vi "MICSD Wakeup RSSI.vi"(8 "error in":errorcluster, 9 "# of Average Points (20)":i32=20, 10 "RSSI Mode (Single)":enum16{"Single Reading", "Average, 20 Rdngs"}(ring), 11 "VISA Resource Name":refnum<visa-resource-name>) -> (0 "error out":errorcluster, 2 "Wakeup RSSI":i16, 3 "dup VISA Resource Name":refnum<visa-resource-name>)   [LabVIEW 2020]
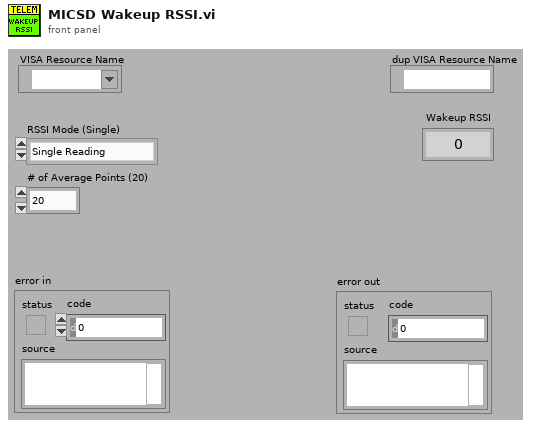
[diagram p1: front panel]
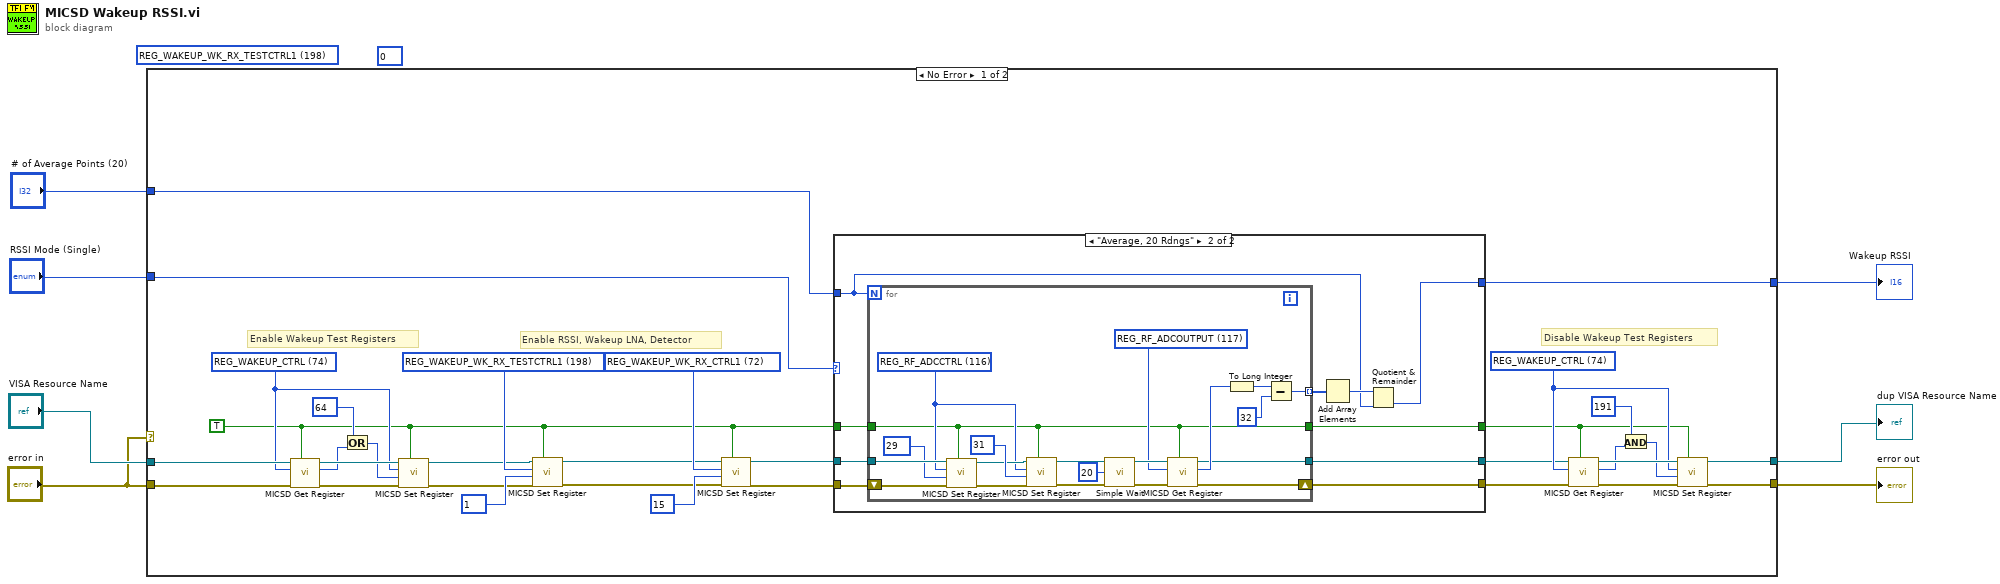
[diagram p0: block diagram]
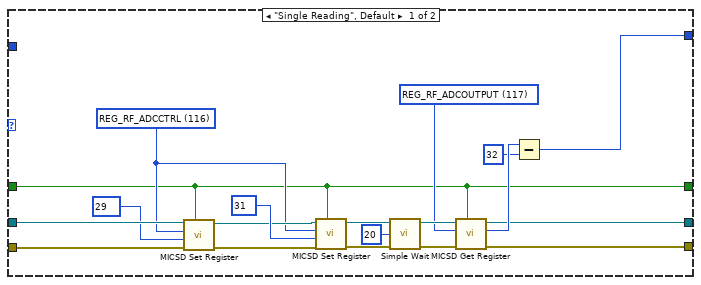
[diagram p2: hidden frame]
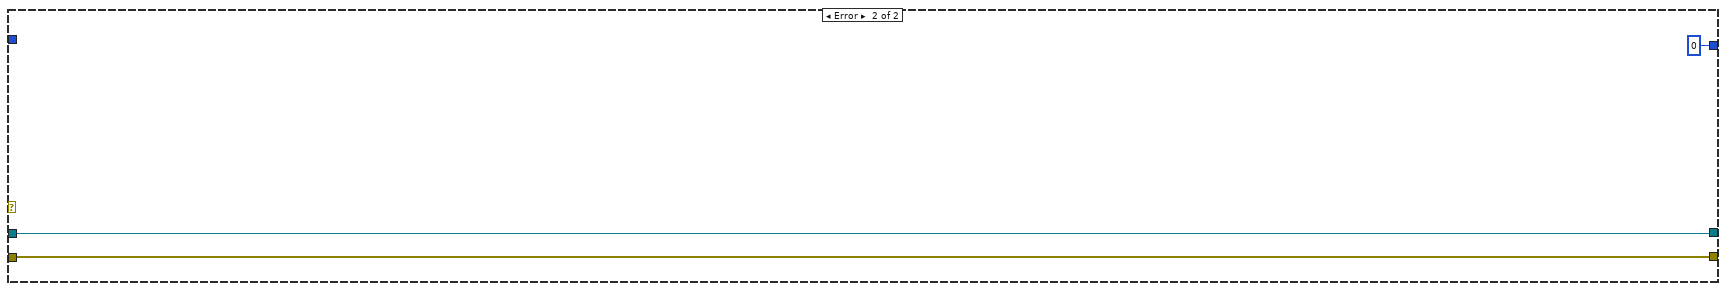
[diagram p3: hidden frame]
diagram:
  (unwired) u16 198 items=["---MANUAL ENTRY---"=1000, "REG_NOREG"=0, "REG_RXBUFF_USED"=1, "REG_RXBUFF_BSIZE"=2, "REG_TXBUFF_USED"=3, "REG_TXBUFF_BSIZE"=4, "REG_TXBUFF_MAXPACKSIZE"=5, "REG_MAC_ERRCLR"=6, "REG_MAC_TRAINNUM"=7, "REG_MAC_SYNCMATCH"=8, "REG_MAC_SYNC1"=9, "REG_MAC_SYNC2"=10, "REG_MAC_SYNC3"=11, "REG_MAC_SYNC4"=12, "REG_MAC_SYNC5"=13, "REG_MAC_MAXBERR"=14, "REG_MAC_ECCORR"=15, "REG_MAC_CRCERR"=16, "REG_MAC_BLKCNT1"=17, "REG_MAC_BLKCNT2"=18, "REG_MAC_IMDTRANSID1"=19, "REG_MAC_IMDTRANSID2"=20, "REG_MAC_IMDTRANSID3"=21, "REG_MAC_COMPANYID"=22, "REG_MAC_MODUSER"=23, "REG_MAC_CHANNEL"=25, "REG_MAC_CLEARWDOG"=26, "REG_MAC_CKCORRTHRESH"=27, "REG_HK_TXADDR"=28, "REG_HK_TXDATA"=29, "REG_HK_TXREPLY"=30, "REG_HK_USERDATA"=31, "REG_HK_USERSTATUS"=32, "REG_HK_LASTADDRESS"=33, "REG_HK_MODE"=34, "REG_MAC_STATUSSEQ"=35, "REG_MAC_MAXRETRIES"=36, "REG_MAC_RESENDTIME"=37, "REG_MAC_POWERSAVETIME"=38, "REG_MAC_HEAD_DET"=39, "REG_MAC_CTRL"=41, "REG_MAC_INITCOM"=42, "REG_INTERFACE_MODE"=43, "REG_TXRXBUFF_BOTH"=44, "REG_TXRXBUFF"=45, "REG_IRQ_RAWSTATUS1"=46, "REG_IRQ_ENABLE1"=47, "REG_IRQ_ENABLESET1"=48, "REG_IRQ_ENABLECLEAR1"=49, "REG_IRQ_RAWSTATUS2"=50, "REG_IRQ_ENABLE2"=51, "REG_IRQ_ENABLESET2"=52, "REG_IRQ_ENABLECLEAR2"=53, "REG_IRQ_STATUS1"=54, "REG_IRQ_STATUS2"=55, "REG_IRQ_AUXSTATUS"=56, "REG_TXBUFF_OVERFLOW"=57, "REG_PO0"=58, "REG_P01"=59, "REG_P02"=60, "REG_P03"=61, "REG_GP0"=62, "REG_GPI"=63, "REG_WAKEUP_245IN"=64, "REG_WAKEUP_COMPANYID"=65, "REG_WAKEUP_IMDTRANSID1"=66, "REG_WAKEUP_IMDTRANSID2"=67, "REG_WAKEUP_IMDTRANSID3"=68, "REG_WAKEUP_CHANNEL"=69, "REG_WAKEUP_MODUSER"=70, "REG_WAKEUP_DEVICEMODE"=71, "REG_WAKEUP_WK_RX_CTRL1"=72, "REG_WAKEUP_STACK_ADDR"=73, "REG_WAKEUP_CTRL"=74, "REG_WAKEUP_STROSCRTRIM"=75, "REG_WAKEUP_BIASTRIM"=76, "REG_WAKEUP_ANT245TUNE"=77, "REG_WAKEUP_WK_RX_RTRIMDET"=78, "REG_WAKEUP_WK_RX_RTRIMDEMOD"=79, "REG_WAKEUP_WK_RX_RSSIGAIN"=80, "REG_WAKEUP_LNAFREQ1"=81, "REG_WAKEUP_STACK"=83, "REG_WAKUP_XOSU"=84, "REG_WAKUP_CNTDROPOUT"=85, "REG_WAKEUP_CRCCTRL"=86, "REG_WAKEUP_CRCWORD1"=87, "REG_WAKEUP_CRCWORD2"=88, "REG_WAKEUP_WK_RX_CTRIM"=89, "REG_WAKEUP_VDDATRIM"=90, "REG_WAKEUP_VDDDTRIM"=91, "REG_WAKEUP_TESTIOBUFEN"=92, "REG_WAKEUP_TESTIOCLAMP"=93, "CORE_RESET_ADDRESS"=94, "CHIP_RESET_ADDRESS"=95, "REG_RF_TXGENCTRL"=96, "REG_RF_TXIFCTRL"=97, "REG_RF_TXRF_SEL_CTRL"=98, "REG_RF_TXRFPWRDEFAULTSET"=99, "REG_RF_RSSITRIM"=100, "REG_RF_TXIFOSCTUNE"=101, "REG_RF_TXIFGAINIMB"=102, "REG_RF_TXIFLOCK"=103, "REG_RF_RXRFLNAGAINTRIM"=104, "REG_RF_RXBIASTR"=105, "REG_RF_RXGENCTRL"=106, "REG_RF_RXIFADCDECLEV"=107, "REG_RF_RXIFDETFILTERTUNE"=108, "REG_RF_RXIFFILTERTUNE"=109, "REG_RF_GENENABLES"=110, "REG_RF_SYNTH_CHANNEL"=111, "REG_TX_RAMP_RTRIM"=112, "REG_TX_RAMP_CTRIM"=113, "REG_RF_XO_TRIM"=114, "REG_RF_SYNTH_SET_TRIM"=115, "REG_RF_ADCCTRL"=116, "REG_RF_ADCOUTPUT"=117, "REG_RF_TXIFAMP"=118, "REG_RF_SYNTH_RTRIM"=119, "REG_RF_SYNTH_CTRIM"=120, "REG_RF_SYNTH_CT"=121, "REG_RF_TXMIXER_IOSTRIM_HIGH_IP"=122, "REG_RF_TXMIXER_IOSTRIM_HIGH_IN"=123, "REG_RF_TXMIXER_IOSTRIM_HIGH_QP"=124, "REG_RF_TXMIXER_IOSTRIM_HIGH_QN"=125, "REG_HX_WUADDR"=126, "REG_REVISION"=127, "REG_NOREG_TEST"=128, "REG_DTEST_RXBUFF"=129, "REG_RXBUFF_NEXT_BLOCK"=130, "REG_RXBUFF_FIRST_IN_PACK"=131, "REG_RXBUFF_FIRST_EMPTY"=132, "REG_MAC_BYPASS"=133, "REG_DTEST_TXBUFF"=134, "REG_TXBUFF_NEXT_BLOCK"=135, "REG_TXBUFF_FIRST_IN_PACK"=136, "REG_TXBUFF_FIRST_EMPTY"=137, "REG_DTEST_SEQ"=138, "REG_DTEST_CKCORR"=139, "REG_MAC_TOPSTATE"=140, "REG_DTEST_INTERFACE"=141, "REG_IFACE_TXRX_BYPASS"=142, "REG_MAC_TXRXWAIT"=143, "REG_MAC_TXRFRAMP"=144, "REG_MAC_TRAINWORD"=145, "REG_MAC_TRAINWORD2"=146, "REG_MAC_SETTINGS"=147, "REG_MAC_CALSELECT1"=148, "REG_MAC_CALSELECT2"=149, "REG_MAC_ANTMATCHSEL"=150, "REG_MAC_ANTTUNESEL1"=151, "REG_MAC_ANTTUNESEL2"=152, "REG_MAC_ANTTUNESEL3"=153, "REG_MAC_ANTTUNESTEP"=154, "REG_MAC_WUMODEBURST"=156, "REG_MAC_WUOFFSHORT"=157, "REG_MAC_WUOFFLONG"=158, "REG_MAC_CLKRECCTRL"=159, "REG_HK_MODE_P2"=162, "REG_MAC_ANTTUNERES1"=164, "REG_MAC_ANTTUNERES2"=165, "REG_INTERFACE_MODE_TEST"=171, "REG_TXRXBUFF_BOTH_P2"=172, "REG_TXRXBUFF_P2"=173, "REG_IRQ_RAWSTATUS1_P2"=174, "REG_MAC_TXIFSTATUS1"=176, "REG_MAC_TXIFSTATUS2"=177, "REG_IRQ_RAWSTATUS2_P2"=178, "REG_MAC_TXIFRAMPDELAY"=179, "REG_MAC_TXIFRAMPSLOPE"=180, "REG_MAX_TXIFRAMP"=181, "REG_IRQ_STATUS1_P2"=182, "REG_IRQ_STATUS2_P2"=183, "REG_IRQ_AUXSTATUS_P2"=184, "REG_MAC_UNLOCK"=188, "REG_MAC_TXIFFREQ"=190, "REG_WAKEUP_TESTCTRL1"=192, "REG_WAKEUP_RX_EN_CNT"=193, "REG_WAKEUP_TESTENABLES"=194, "REG_WAKEUP_DTBI_CTRL"=195, "REG_WAKEUP_DTBO_CTRL"=196, "REG_WAKEUP_TESTIOBUFTEST"=197, "REG_WAKEUP_WK_RX_TESTCTRL1"=198, "REG_WAKEUP_WK_RX_TESTCTRL2"=199, "REG_WAKEUP_SENS_SEQUENCE_CTRL"=200, "REG_WAKEUP_LNABIAS"=201, "REG_WAKEUP_DET_TH_TRIM1"=202, "REG_WAKEUP_LNABIAS_NOM1"=203, "REG_WAKEUP_RX_TSHORT_TRIM1"=204, "REG_WAKEUP_LNABIAS_NOM2"=205, "REG_WAKEUP_RX_TLONG_TRIM1"=206, "REG_WAKEUP_LNA_NEGRTRIM_NOM1"=207, "REG_WAKEUP_RX_TBURST_TRIM1"=208, "REG_WAKEUP_RX_LNA_NEGRTRIM_NOM2"=209, "REG_WAKEUP_RX_BB_G_BW_SEL1"=210, "REG_WAKEUP_WK_RX_DET_IOSTRIM1"=212, "REG_WAKEUP_WK_RX_CTRL2"=214, "REG_WAKEUP_WK_RX_RSSIVOSTRIM"=215, "REG_WAKEUP_LNANEGR_EFF"=216, "REG_WAKEUP_XOSU_FAST"=217, "REG_WAKEUP_STROSCPWIDTH1"=218, "REG_WAKEUP_STROSCPERIOD1"=220, "REG_WAKEUP_STROSCPERIOD2"=221, "REG_WAKEUP_WK_RX_LNA_NEGRTRIM1"=222, "REG_RF_TXTESTENABLE"=224, "REG_RF_TXIFTESTMODE"=225, "REG_RF_RXTESTENABLE"=226, "REG_RF_RXIFTESTCTRL1"=227, "REG_RF_RXIFTESTCTRL2"=228, "REG_RF_RXIFTESTCTRL3"=229, "REG_RF_SYNTH_TESTCTRL1"=230, "REG_RF_SYNTH_TESTCTRL2"=231, "REG_RF_SYNTH_TESTCTRL3"=232, "REG_RF_ADCTEST1"=237, "REG_RF_ADCTEST2"=238, "REG_RF_TXMIXER_IOSTRIM_LOW_IP"=240, "REG_RF_TXMIXER_IOSTRIM_LOW_IN"=241, "REG_RF_TXMIXER_ISOTRIM_LOW_QP"=242, "REG_RF_TXMIXER_IOSTRIM_LOW_QN"=243, "REG_RF_SYNTH_KPD"=244, "REG_RF_SYNTH_LOLEV"=245, "REG_RF_TXRFPWRTUNEANTSET"=246, "REG_RF_TXPD_GAIN_CTRL"=247, "REG_RF_SYNTH_STARTUP"=248, "REG_RF_TXRFANTTUNE_TXMODE"=249, "REG_RF_TXRFANTTUNE_RXMODE"=250, "REG_RF_RXRFANTTUNE_TXMODE"=251, "REG_RF_RXRFANTTUNE_RXMODE"=252, "REG_ANTMATCH1"=253, "REG_ANTMATCH2"=254, "REG_REVISION_P2"=255] ("Register")
  (unwired) u8 0 ("Data")
  n1 = case shown="No Error" "error in" {
    tunnel: "VISA Resource Name" -> [w40 w90]
    tunnel: "error in" -> [w39 w89]
    tunnel: [w14 w89] -> w6
    tunnel: [w13 w90] -> w5
    tunnel: "RSSI Mode (Single)" -> [w11 _]
    tunnel: "# of Average Points (20)" -> [w9 _]
    tunnel: [w8 0] -> w1
    frame No Error {
      w12 = TRUE
      w15 = u16 74 items=["---MANUAL ENTRY---"=1000, "REG_NOREG"=0, "REG_RXBUFF_USED"=1, "REG_RXBUFF_BSIZE"=2, "REG_TXBUFF_USED"=3, "REG_TXBUFF_BSIZE"=4, "REG_TXBUFF_MAXPACKSIZE"=5, "REG_MAC_ERRCLR"=6, "REG_MAC_TRAINNUM"=7, "REG_MAC_SYNCMATCH"=8, "REG_MAC_SYNC1"=9, "REG_MAC_SYNC2"=10, "REG_MAC_SYNC3"=11, "REG_MAC_SYNC4"=12, "REG_MAC_SYNC5"=13, "REG_MAC_MAXBERR"=14, "REG_MAC_ECCORR"=15, "REG_MAC_CRCERR"=16, "REG_MAC_BLKCNT1"=17, "REG_MAC_BLKCNT2"=18, "REG_MAC_IMDTRANSID1"=19, "REG_MAC_IMDTRANSID2"=20, "REG_MAC_IMDTRANSID3"=21, "REG_MAC_COMPANYID"=22, "REG_MAC_MODUSER"=23, "REG_MAC_CHANNEL"=25, "REG_MAC_CLEARWDOG"=26, "REG_MAC_CKCORRTHRESH"=27, "REG_HK_TXADDR"=28, "REG_HK_TXDATA"=29, "REG_HK_TXREPLY"=30, "REG_HK_USERDATA"=31, "REG_HK_USERSTATUS"=32, "REG_HK_LASTADDRESS"=33, "REG_HK_MODE"=34, "REG_MAC_STATUSSEQ"=35, "REG_MAC_MAXRETRIES"=36, "REG_MAC_RESENDTIME"=37, "REG_MAC_POWERSAVETIME"=38, "REG_MAC_HEAD_DET"=39, "REG_MAC_CTRL"=41, "REG_MAC_INITCOM"=42, "REG_INTERFACE_MODE"=43, "REG_TXRXBUFF_BOTH"=44, "REG_TXRXBUFF"=45, "REG_IRQ_RAWSTATUS1"=46, "REG_IRQ_ENABLE1"=47, "REG_IRQ_ENABLESET1"=48, "REG_IRQ_ENABLECLEAR1"=49, "REG_IRQ_RAWSTATUS2"=50, "REG_IRQ_ENABLE2"=51, "REG_IRQ_ENABLESET2"=52, "REG_IRQ_ENABLECLEAR2"=53, "REG_IRQ_STATUS1"=54, "REG_IRQ_STATUS2"=55, "REG_IRQ_AUXSTATUS"=56, "REG_TXBUFF_OVERFLOW"=57, "REG_PO0"=58, "REG_P01"=59, "REG_P02"=60, "REG_P03"=61, "REG_GP0"=62, "REG_GPI"=63, "REG_WAKEUP_245IN"=64, "REG_WAKEUP_COMPANYID"=65, "REG_WAKEUP_IMDTRANSID1"=66, "REG_WAKEUP_IMDTRANSID2"=67, "REG_WAKEUP_IMDTRANSID3"=68, "REG_WAKEUP_CHANNEL"=69, "REG_WAKEUP_MODUSER"=70, "REG_WAKEUP_DEVICEMODE"=71, "REG_WAKEUP_WK_RX_CTRL1"=72, "REG_WAKEUP_STACK_ADDR"=73, "REG_WAKEUP_CTRL"=74, "REG_WAKEUP_STROSCRTRIM"=75, "REG_WAKEUP_BIASTRIM"=76, "REG_WAKEUP_ANT245TUNE"=77, "REG_WAKEUP_WK_RX_RTRIMDET"=78, "REG_WAKEUP_WK_RX_RTRIMDEMOD"=79, "REG_WAKEUP_WK_RX_RSSIGAIN"=80, "REG_WAKEUP_LNAFREQ1"=81, "REG_WAKEUP_STACK"=83, "REG_WAKUP_XOSU"=84, "REG_WAKUP_CNTDROPOUT"=85, "REG_WAKEUP_CRCCTRL"=86, "REG_WAKEUP_CRCWORD1"=87, "REG_WAKEUP_CRCWORD2"=88, "REG_WAKEUP_WK_RX_CTRIM"=89, "REG_WAKEUP_VDDATRIM"=90, "REG_WAKEUP_VDDDTRIM"=91, "REG_WAKEUP_TESTIOBUFEN"=92, "REG_WAKEUP_TESTIOCLAMP"=93, "CORE_RESET_ADDRESS"=94, "CHIP_RESET_ADDRESS"=95, "REG_RF_TXGENCTRL"=96, "REG_RF_TXIFCTRL"=97, "REG_RF_TXRF_SEL_CTRL"=98, "REG_RF_TXRFPWRDEFAULTSET"=99, "REG_RF_RSSITRIM"=100, "REG_RF_TXIFOSCTUNE"=101, "REG_RF_TXIFGAINIMB"=102, "REG_RF_TXIFLOCK"=103, "REG_RF_RXRFLNAGAINTRIM"=104, "REG_RF_RXBIASTR"=105, "REG_RF_RXGENCTRL"=106, "REG_RF_RXIFADCDECLEV"=107, "REG_RF_RXIFDETFILTERTUNE"=108, "REG_RF_RXIFFILTERTUNE"=109, "REG_RF_GENENABLES"=110, "REG_RF_SYNTH_CHANNEL"=111, "REG_TX_RAMP_RTRIM"=112, "REG_TX_RAMP_CTRIM"=113, "REG_RF_XO_TRIM"=114, "REG_RF_SYNTH_SET_TRIM"=115, "REG_RF_ADCCTRL"=116, "REG_RF_ADCOUTPUT"=117, "REG_RF_TXIFAMP"=118, "REG_RF_SYNTH_RTRIM"=119, "REG_RF_SYNTH_CTRIM"=120, "REG_RF_SYNTH_CT"=121, "REG_RF_TXMIXER_IOSTRIM_HIGH_IP"=122, "REG_RF_TXMIXER_IOSTRIM_HIGH_IN"=123, "REG_RF_TXMIXER_IOSTRIM_HIGH_QP"=124, "REG_RF_TXMIXER_IOSTRIM_HIGH_QN"=125, "REG_HX_WUADDR"=126, "REG_REVISION"=127, "REG_NOREG_TEST"=128, "REG_DTEST_RXBUFF"=129, "REG_RXBUFF_NEXT_BLOCK"=130, "REG_RXBUFF_FIRST_IN_PACK"=131, "REG_RXBUFF_FIRST_EMPTY"=132, "REG_MAC_BYPASS"=133, "REG_DTEST_TXBUFF"=134, "REG_TXBUFF_NEXT_BLOCK"=135, "REG_TXBUFF_FIRST_IN_PACK"=136, "REG_TXBUFF_FIRST_EMPTY"=137, "REG_DTEST_SEQ"=138, "REG_DTEST_CKCORR"=139, "REG_MAC_TOPSTATE"=140, "REG_DTEST_INTERFACE"=141, "REG_IFACE_TXRX_BYPASS"=142, "REG_MAC_TXRXWAIT"=143, "REG_MAC_TXRFRAMP"=144, "REG_MAC_TRAINWORD"=145, "REG_MAC_TRAINWORD2"=146, "REG_MAC_SETTINGS"=147, "REG_MAC_CALSELECT1"=148, "REG_MAC_CALSELECT2"=149, "REG_MAC_ANTMATCHSEL"=150, "REG_MAC_ANTTUNESEL1"=151, "REG_MAC_ANTTUNESEL2"=152, "REG_MAC_ANTTUNESEL3"=153, "REG_MAC_ANTTUNESTEP"=154, "REG_MAC_WUMODEBURST"=156, "REG_MAC_WUOFFSHORT"=157, "REG_MAC_WUOFFLONG"=158, "REG_MAC_CLKRECCTRL"=159, "REG_HK_MODE_P2"=162, "REG_MAC_ANTTUNERES1"=164, "REG_MAC_ANTTUNERES2"=165, "REG_INTERFACE_MODE_TEST"=171, "REG_TXRXBUFF_BOTH_P2"=172, "REG_TXRXBUFF_P2"=173, "REG_IRQ_RAWSTATUS1_P2"=174, "REG_MAC_TXIFSTATUS1"=176, "REG_MAC_TXIFSTATUS2"=177, "REG_IRQ_RAWSTATUS2_P2"=178, "REG_MAC_TXIFRAMPDELAY"=179, "REG_MAC_TXIFRAMPSLOPE"=180, "REG_MAX_TXIFRAMP"=181, "REG_IRQ_STATUS1_P2"=182, "REG_IRQ_STATUS2_P2"=183, "REG_IRQ_AUXSTATUS_P2"=184, "REG_MAC_UNLOCK"=188, "REG_MAC_TXIFFREQ"=190, "REG_WAKEUP_TESTCTRL1"=192, "REG_WAKEUP_RX_EN_CNT"=193, "REG_WAKEUP_TESTENABLES"=194, "REG_WAKEUP_DTBI_CTRL"=195, "REG_WAKEUP_DTBO_CTRL"=196, "REG_WAKEUP_TESTIOBUFTEST"=197, "REG_WAKEUP_WK_RX_TESTCTRL1"=198, "REG_WAKEUP_WK_RX_TESTCTRL2"=199, "REG_WAKEUP_SENS_SEQUENCE_CTRL"=200, "REG_WAKEUP_LNABIAS"=201, "REG_WAKEUP_DET_TH_TRIM1"=202, "REG_WAKEUP_LNABIAS_NOM1"=203, "REG_WAKEUP_RX_TSHORT_TRIM1"=204, "REG_WAKEUP_LNABIAS_NOM2"=205, "REG_WAKEUP_RX_TLONG_TRIM1"=206, "REG_WAKEUP_LNA_NEGRTRIM_NOM1"=207, "REG_WAKEUP_RX_TBURST_TRIM1"=208, "REG_WAKEUP_RX_LNA_NEGRTRIM_NOM2"=209, "REG_WAKEUP_RX_BB_G_BW_SEL1"=210, "REG_WAKEUP_WK_RX_DET_IOSTRIM1"=212, "REG_WAKEUP_WK_RX_CTRL2"=214, "REG_WAKEUP_WK_RX_RSSIVOSTRIM"=215, "REG_WAKEUP_LNANEGR_EFF"=216, "REG_WAKEUP_XOSU_FAST"=217, "REG_WAKEUP_STROSCPWIDTH1"=218, "REG_WAKEUP_STROSCPERIOD1"=220, "REG_WAKEUP_STROSCPERIOD2"=221, "REG_WAKEUP_WK_RX_LNA_NEGRTRIM1"=222, "REG_RF_TXTESTENABLE"=224, "REG_RF_TXIFTESTMODE"=225, "REG_RF_RXTESTENABLE"=226, "REG_RF_RXIFTESTCTRL1"=227, "REG_RF_RXIFTESTCTRL2"=228, "REG_RF_RXIFTESTCTRL3"=229, "REG_RF_SYNTH_TESTCTRL1"=230, "REG_RF_SYNTH_TESTCTRL2"=231, "REG_RF_SYNTH_TESTCTRL3"=232, "REG_RF_ADCTEST1"=237, "REG_RF_ADCTEST2"=238, "REG_RF_TXMIXER_IOSTRIM_LOW_IP"=240, "REG_RF_TXMIXER_IOSTRIM_LOW_IN"=241, "REG_RF_TXMIXER_ISOTRIM_LOW_QP"=242, "REG_RF_TXMIXER_IOSTRIM_LOW_QN"=243, "REG_RF_SYNTH_KPD"=244, "REG_RF_SYNTH_LOLEV"=245, "REG_RF_TXRFPWRTUNEANTSET"=246, "REG_RF_TXPD_GAIN_CTRL"=247, "REG_RF_SYNTH_STARTUP"=248, "REG_RF_TXRFANTTUNE_TXMODE"=249, "REG_RF_TXRFANTTUNE_RXMODE"=250, "REG_RF_RXRFANTTUNE_TXMODE"=251, "REG_RF_RXRFANTTUNE_RXMODE"=252, "REG_ANTMATCH1"=253, "REG_ANTMATCH2"=254, "REG_REVISION_P2"=255] ("Register")
      w26 = u16 72 items=["---MANUAL ENTRY---"=1000, "REG_NOREG"=0, "REG_RXBUFF_USED"=1, "REG_RXBUFF_BSIZE"=2, "REG_TXBUFF_USED"=3, "REG_TXBUFF_BSIZE"=4, "REG_TXBUFF_MAXPACKSIZE"=5, "REG_MAC_ERRCLR"=6, "REG_MAC_TRAINNUM"=7, "REG_MAC_SYNCMATCH"=8, "REG_MAC_SYNC1"=9, "REG_MAC_SYNC2"=10, "REG_MAC_SYNC3"=11, "REG_MAC_SYNC4"=12, "REG_MAC_SYNC5"=13, "REG_MAC_MAXBERR"=14, "REG_MAC_ECCORR"=15, "REG_MAC_CRCERR"=16, "REG_MAC_BLKCNT1"=17, "REG_MAC_BLKCNT2"=18, "REG_MAC_IMDTRANSID1"=19, "REG_MAC_IMDTRANSID2"=20, "REG_MAC_IMDTRANSID3"=21, "REG_MAC_COMPANYID"=22, "REG_MAC_MODUSER"=23, "REG_MAC_CHANNEL"=25, "REG_MAC_CLEARWDOG"=26, "REG_MAC_CKCORRTHRESH"=27, "REG_HK_TXADDR"=28, "REG_HK_TXDATA"=29, "REG_HK_TXREPLY"=30, "REG_HK_USERDATA"=31, "REG_HK_USERSTATUS"=32, "REG_HK_LASTADDRESS"=33, "REG_HK_MODE"=34, "REG_MAC_STATUSSEQ"=35, "REG_MAC_MAXRETRIES"=36, "REG_MAC_RESENDTIME"=37, "REG_MAC_POWERSAVETIME"=38, "REG_MAC_HEAD_DET"=39, "REG_MAC_CTRL"=41, "REG_MAC_INITCOM"=42, "REG_INTERFACE_MODE"=43, "REG_TXRXBUFF_BOTH"=44, "REG_TXRXBUFF"=45, "REG_IRQ_RAWSTATUS1"=46, "REG_IRQ_ENABLE1"=47, "REG_IRQ_ENABLESET1"=48, "REG_IRQ_ENABLECLEAR1"=49, "REG_IRQ_RAWSTATUS2"=50, "REG_IRQ_ENABLE2"=51, "REG_IRQ_ENABLESET2"=52, "REG_IRQ_ENABLECLEAR2"=53, "REG_IRQ_STATUS1"=54, "REG_IRQ_STATUS2"=55, "REG_IRQ_AUXSTATUS"=56, "REG_TXBUFF_OVERFLOW"=57, "REG_PO0"=58, "REG_P01"=59, "REG_P02"=60, "REG_P03"=61, "REG_GP0"=62, "REG_GPI"=63, "REG_WAKEUP_245IN"=64, "REG_WAKEUP_COMPANYID"=65, "REG_WAKEUP_IMDTRANSID1"=66, "REG_WAKEUP_IMDTRANSID2"=67, "REG_WAKEUP_IMDTRANSID3"=68, "REG_WAKEUP_CHANNEL"=69, "REG_WAKEUP_MODUSER"=70, "REG_WAKEUP_DEVICEMODE"=71, "REG_WAKEUP_WK_RX_CTRL1"=72, "REG_WAKEUP_STACK_ADDR"=73, "REG_WAKEUP_CTRL"=74, "REG_WAKEUP_STROSCRTRIM"=75, "REG_WAKEUP_BIASTRIM"=76, "REG_WAKEUP_ANT245TUNE"=77, "REG_WAKEUP_WK_RX_RTRIMDET"=78, "REG_WAKEUP_WK_RX_RTRIMDEMOD"=79, "REG_WAKEUP_WK_RX_RSSIGAIN"=80, "REG_WAKEUP_LNAFREQ1"=81, "REG_WAKEUP_STACK"=83, "REG_WAKUP_XOSU"=84, "REG_WAKUP_CNTDROPOUT"=85, "REG_WAKEUP_CRCCTRL"=86, "REG_WAKEUP_CRCWORD1"=87, "REG_WAKEUP_CRCWORD2"=88, "REG_WAKEUP_WK_RX_CTRIM"=89, "REG_WAKEUP_VDDATRIM"=90, "REG_WAKEUP_VDDDTRIM"=91, "REG_WAKEUP_TESTIOBUFEN"=92, "REG_WAKEUP_TESTIOCLAMP"=93, "CORE_RESET_ADDRESS"=94, "CHIP_RESET_ADDRESS"=95, "REG_RF_TXGENCTRL"=96, "REG_RF_TXIFCTRL"=97, "REG_RF_TXRF_SEL_CTRL"=98, "REG_RF_TXRFPWRDEFAULTSET"=99, "REG_RF_RSSITRIM"=100, "REG_RF_TXIFOSCTUNE"=101, "REG_RF_TXIFGAINIMB"=102, "REG_RF_TXIFLOCK"=103, "REG_RF_RXRFLNAGAINTRIM"=104, "REG_RF_RXBIASTR"=105, "REG_RF_RXGENCTRL"=106, "REG_RF_RXIFADCDECLEV"=107, "REG_RF_RXIFDETFILTERTUNE"=108, "REG_RF_RXIFFILTERTUNE"=109, "REG_RF_GENENABLES"=110, "REG_RF_SYNTH_CHANNEL"=111, "REG_TX_RAMP_RTRIM"=112, "REG_TX_RAMP_CTRIM"=113, "REG_RF_XO_TRIM"=114, "REG_RF_SYNTH_SET_TRIM"=115, "REG_RF_ADCCTRL"=116, "REG_RF_ADCOUTPUT"=117, "REG_RF_TXIFAMP"=118, "REG_RF_SYNTH_RTRIM"=119, "REG_RF_SYNTH_CTRIM"=120, "REG_RF_SYNTH_CT"=121, "REG_RF_TXMIXER_IOSTRIM_HIGH_IP"=122, "REG_RF_TXMIXER_IOSTRIM_HIGH_IN"=123, "REG_RF_TXMIXER_IOSTRIM_HIGH_QP"=124, "REG_RF_TXMIXER_IOSTRIM_HIGH_QN"=125, "REG_HX_WUADDR"=126, "REG_REVISION"=127, "REG_NOREG_TEST"=128, "REG_DTEST_RXBUFF"=129, "REG_RXBUFF_NEXT_BLOCK"=130, "REG_RXBUFF_FIRST_IN_PACK"=131, "REG_RXBUFF_FIRST_EMPTY"=132, "REG_MAC_BYPASS"=133, "REG_DTEST_TXBUFF"=134, "REG_TXBUFF_NEXT_BLOCK"=135, "REG_TXBUFF_FIRST_IN_PACK"=136, "REG_TXBUFF_FIRST_EMPTY"=137, "REG_DTEST_SEQ"=138, "REG_DTEST_CKCORR"=139, "REG_MAC_TOPSTATE"=140, "REG_DTEST_INTERFACE"=141, "REG_IFACE_TXRX_BYPASS"=142, "REG_MAC_TXRXWAIT"=143, "REG_MAC_TXRFRAMP"=144, "REG_MAC_TRAINWORD"=145, "REG_MAC_TRAINWORD2"=146, "REG_MAC_SETTINGS"=147, "REG_MAC_CALSELECT1"=148, "REG_MAC_CALSELECT2"=149, "REG_MAC_ANTMATCHSEL"=150, "REG_MAC_ANTTUNESEL1"=151, "REG_MAC_ANTTUNESEL2"=152, "REG_MAC_ANTTUNESEL3"=153, "REG_MAC_ANTTUNESTEP"=154, "REG_MAC_WUMODEBURST"=156, "REG_MAC_WUOFFSHORT"=157, "REG_MAC_WUOFFLONG"=158, "REG_MAC_CLKRECCTRL"=159, "REG_HK_MODE_P2"=162, "REG_MAC_ANTTUNERES1"=164, "REG_MAC_ANTTUNERES2"=165, "REG_INTERFACE_MODE_TEST"=171, "REG_TXRXBUFF_BOTH_P2"=172, "REG_TXRXBUFF_P2"=173, "REG_IRQ_RAWSTATUS1_P2"=174, "REG_MAC_TXIFSTATUS1"=176, "REG_MAC_TXIFSTATUS2"=177, "REG_IRQ_RAWSTATUS2_P2"=178, "REG_MAC_TXIFRAMPDELAY"=179, "REG_MAC_TXIFRAMPSLOPE"=180, "REG_MAX_TXIFRAMP"=181, "REG_IRQ_STATUS1_P2"=182, "REG_IRQ_STATUS2_P2"=183, "REG_IRQ_AUXSTATUS_P2"=184, "REG_MAC_UNLOCK"=188, "REG_MAC_TXIFFREQ"=190, "REG_WAKEUP_TESTCTRL1"=192, "REG_WAKEUP_RX_EN_CNT"=193, "REG_WAKEUP_TESTENABLES"=194, "REG_WAKEUP_DTBI_CTRL"=195, "REG_WAKEUP_DTBO_CTRL"=196, "REG_WAKEUP_TESTIOBUFTEST"=197, "REG_WAKEUP_WK_RX_TESTCTRL1"=198, "REG_WAKEUP_WK_RX_TESTCTRL2"=199, "REG_WAKEUP_SENS_SEQUENCE_CTRL"=200, "REG_WAKEUP_LNABIAS"=201, "REG_WAKEUP_DET_TH_TRIM1"=202, "REG_WAKEUP_LNABIAS_NOM1"=203, "REG_WAKEUP_RX_TSHORT_TRIM1"=204, "REG_WAKEUP_LNABIAS_NOM2"=205, "REG_WAKEUP_RX_TLONG_TRIM1"=206, "REG_WAKEUP_LNA_NEGRTRIM_NOM1"=207, "REG_WAKEUP_RX_TBURST_TRIM1"=208, "REG_WAKEUP_RX_LNA_NEGRTRIM_NOM2"=209, "REG_WAKEUP_RX_BB_G_BW_SEL1"=210, "REG_WAKEUP_WK_RX_DET_IOSTRIM1"=212, "REG_WAKEUP_WK_RX_CTRL2"=214, "REG_WAKEUP_WK_RX_RSSIVOSTRIM"=215, "REG_WAKEUP_LNANEGR_EFF"=216, "REG_WAKEUP_XOSU_FAST"=217, "REG_WAKEUP_STROSCPWIDTH1"=218, "REG_WAKEUP_STROSCPERIOD1"=220, "REG_WAKEUP_STROSCPERIOD2"=221, "REG_WAKEUP_WK_RX_LNA_NEGRTRIM1"=222, "REG_RF_TXTESTENABLE"=224, "REG_RF_TXIFTESTMODE"=225, "REG_RF_RXTESTENABLE"=226, "REG_RF_RXIFTESTCTRL1"=227, "REG_RF_RXIFTESTCTRL2"=228, "REG_RF_RXIFTESTCTRL3"=229, "REG_RF_SYNTH_TESTCTRL1"=230, "REG_RF_SYNTH_TESTCTRL2"=231, "REG_RF_SYNTH_TESTCTRL3"=232, "REG_RF_ADCTEST1"=237, "REG_RF_ADCTEST2"=238, "REG_RF_TXMIXER_IOSTRIM_LOW_IP"=240, "REG_RF_TXMIXER_IOSTRIM_LOW_IN"=241, "REG_RF_TXMIXER_ISOTRIM_LOW_QP"=242, "REG_RF_TXMIXER_IOSTRIM_LOW_QN"=243, "REG_RF_SYNTH_KPD"=244, "REG_RF_SYNTH_LOLEV"=245, "REG_RF_TXRFPWRTUNEANTSET"=246, "REG_RF_TXPD_GAIN_CTRL"=247, "REG_RF_SYNTH_STARTUP"=248, "REG_RF_TXRFANTTUNE_TXMODE"=249, "REG_RF_TXRFANTTUNE_RXMODE"=250, "REG_RF_RXRFANTTUNE_TXMODE"=251, "REG_RF_RXRFANTTUNE_RXMODE"=252, "REG_ANTMATCH1"=253, "REG_ANTMATCH2"=254, "REG_REVISION_P2"=255] ("Register")
      w28 = u16 198 items=["---MANUAL ENTRY---"=1000, "REG_NOREG"=0, "REG_RXBUFF_USED"=1, "REG_RXBUFF_BSIZE"=2, "REG_TXBUFF_USED"=3, "REG_TXBUFF_BSIZE"=4, "REG_TXBUFF_MAXPACKSIZE"=5, "REG_MAC_ERRCLR"=6, "REG_MAC_TRAINNUM"=7, "REG_MAC_SYNCMATCH"=8, "REG_MAC_SYNC1"=9, "REG_MAC_SYNC2"=10, "REG_MAC_SYNC3"=11, "REG_MAC_SYNC4"=12, "REG_MAC_SYNC5"=13, "REG_MAC_MAXBERR"=14, "REG_MAC_ECCORR"=15, "REG_MAC_CRCERR"=16, "REG_MAC_BLKCNT1"=17, "REG_MAC_BLKCNT2"=18, "REG_MAC_IMDTRANSID1"=19, "REG_MAC_IMDTRANSID2"=20, "REG_MAC_IMDTRANSID3"=21, "REG_MAC_COMPANYID"=22, "REG_MAC_MODUSER"=23, "REG_MAC_CHANNEL"=25, "REG_MAC_CLEARWDOG"=26, "REG_MAC_CKCORRTHRESH"=27, "REG_HK_TXADDR"=28, "REG_HK_TXDATA"=29, "REG_HK_TXREPLY"=30, "REG_HK_USERDATA"=31, "REG_HK_USERSTATUS"=32, "REG_HK_LASTADDRESS"=33, "REG_HK_MODE"=34, "REG_MAC_STATUSSEQ"=35, "REG_MAC_MAXRETRIES"=36, "REG_MAC_RESENDTIME"=37, "REG_MAC_POWERSAVETIME"=38, "REG_MAC_HEAD_DET"=39, "REG_MAC_CTRL"=41, "REG_MAC_INITCOM"=42, "REG_INTERFACE_MODE"=43, "REG_TXRXBUFF_BOTH"=44, "REG_TXRXBUFF"=45, "REG_IRQ_RAWSTATUS1"=46, "REG_IRQ_ENABLE1"=47, "REG_IRQ_ENABLESET1"=48, "REG_IRQ_ENABLECLEAR1"=49, "REG_IRQ_RAWSTATUS2"=50, "REG_IRQ_ENABLE2"=51, "REG_IRQ_ENABLESET2"=52, "REG_IRQ_ENABLECLEAR2"=53, "REG_IRQ_STATUS1"=54, "REG_IRQ_STATUS2"=55, "REG_IRQ_AUXSTATUS"=56, "REG_TXBUFF_OVERFLOW"=57, "REG_PO0"=58, "REG_P01"=59, "REG_P02"=60, "REG_P03"=61, "REG_GP0"=62, "REG_GPI"=63, "REG_WAKEUP_245IN"=64, "REG_WAKEUP_COMPANYID"=65, "REG_WAKEUP_IMDTRANSID1"=66, "REG_WAKEUP_IMDTRANSID2"=67, "REG_WAKEUP_IMDTRANSID3"=68, "REG_WAKEUP_CHANNEL"=69, "REG_WAKEUP_MODUSER"=70, "REG_WAKEUP_DEVICEMODE"=71, "REG_WAKEUP_WK_RX_CTRL1"=72, "REG_WAKEUP_STACK_ADDR"=73, "REG_WAKEUP_CTRL"=74, "REG_WAKEUP_STROSCRTRIM"=75, "REG_WAKEUP_BIASTRIM"=76, "REG_WAKEUP_ANT245TUNE"=77, "REG_WAKEUP_WK_RX_RTRIMDET"=78, "REG_WAKEUP_WK_RX_RTRIMDEMOD"=79, "REG_WAKEUP_WK_RX_RSSIGAIN"=80, "REG_WAKEUP_LNAFREQ1"=81, "REG_WAKEUP_STACK"=83, "REG_WAKUP_XOSU"=84, "REG_WAKUP_CNTDROPOUT"=85, "REG_WAKEUP_CRCCTRL"=86, "REG_WAKEUP_CRCWORD1"=87, "REG_WAKEUP_CRCWORD2"=88, "REG_WAKEUP_WK_RX_CTRIM"=89, "REG_WAKEUP_VDDATRIM"=90, "REG_WAKEUP_VDDDTRIM"=91, "REG_WAKEUP_TESTIOBUFEN"=92, "REG_WAKEUP_TESTIOCLAMP"=93, "CORE_RESET_ADDRESS"=94, "CHIP_RESET_ADDRESS"=95, "REG_RF_TXGENCTRL"=96, "REG_RF_TXIFCTRL"=97, "REG_RF_TXRF_SEL_CTRL"=98, "REG_RF_TXRFPWRDEFAULTSET"=99, "REG_RF_RSSITRIM"=100, "REG_RF_TXIFOSCTUNE"=101, "REG_RF_TXIFGAINIMB"=102, "REG_RF_TXIFLOCK"=103, "REG_RF_RXRFLNAGAINTRIM"=104, "REG_RF_RXBIASTR"=105, "REG_RF_RXGENCTRL"=106, "REG_RF_RXIFADCDECLEV"=107, "REG_RF_RXIFDETFILTERTUNE"=108, "REG_RF_RXIFFILTERTUNE"=109, "REG_RF_GENENABLES"=110, "REG_RF_SYNTH_CHANNEL"=111, "REG_TX_RAMP_RTRIM"=112, "REG_TX_RAMP_CTRIM"=113, "REG_RF_XO_TRIM"=114, "REG_RF_SYNTH_SET_TRIM"=115, "REG_RF_ADCCTRL"=116, "REG_RF_ADCOUTPUT"=117, "REG_RF_TXIFAMP"=118, "REG_RF_SYNTH_RTRIM"=119, "REG_RF_SYNTH_CTRIM"=120, "REG_RF_SYNTH_CT"=121, "REG_RF_TXMIXER_IOSTRIM_HIGH_IP"=122, "REG_RF_TXMIXER_IOSTRIM_HIGH_IN"=123, "REG_RF_TXMIXER_IOSTRIM_HIGH_QP"=124, "REG_RF_TXMIXER_IOSTRIM_HIGH_QN"=125, "REG_HX_WUADDR"=126, "REG_REVISION"=127, "REG_NOREG_TEST"=128, "REG_DTEST_RXBUFF"=129, "REG_RXBUFF_NEXT_BLOCK"=130, "REG_RXBUFF_FIRST_IN_PACK"=131, "REG_RXBUFF_FIRST_EMPTY"=132, "REG_MAC_BYPASS"=133, "REG_DTEST_TXBUFF"=134, "REG_TXBUFF_NEXT_BLOCK"=135, "REG_TXBUFF_FIRST_IN_PACK"=136, "REG_TXBUFF_FIRST_EMPTY"=137, "REG_DTEST_SEQ"=138, "REG_DTEST_CKCORR"=139, "REG_MAC_TOPSTATE"=140, "REG_DTEST_INTERFACE"=141, "REG_IFACE_TXRX_BYPASS"=142, "REG_MAC_TXRXWAIT"=143, "REG_MAC_TXRFRAMP"=144, "REG_MAC_TRAINWORD"=145, "REG_MAC_TRAINWORD2"=146, "REG_MAC_SETTINGS"=147, "REG_MAC_CALSELECT1"=148, "REG_MAC_CALSELECT2"=149, "REG_MAC_ANTMATCHSEL"=150, "REG_MAC_ANTTUNESEL1"=151, "REG_MAC_ANTTUNESEL2"=152, "REG_MAC_ANTTUNESEL3"=153, "REG_MAC_ANTTUNESTEP"=154, "REG_MAC_WUMODEBURST"=156, "REG_MAC_WUOFFSHORT"=157, "REG_MAC_WUOFFLONG"=158, "REG_MAC_CLKRECCTRL"=159, "REG_HK_MODE_P2"=162, "REG_MAC_ANTTUNERES1"=164, "REG_MAC_ANTTUNERES2"=165, "REG_INTERFACE_MODE_TEST"=171, "REG_TXRXBUFF_BOTH_P2"=172, "REG_TXRXBUFF_P2"=173, "REG_IRQ_RAWSTATUS1_P2"=174, "REG_MAC_TXIFSTATUS1"=176, "REG_MAC_TXIFSTATUS2"=177, "REG_IRQ_RAWSTATUS2_P2"=178, "REG_MAC_TXIFRAMPDELAY"=179, "REG_MAC_TXIFRAMPSLOPE"=180, "REG_MAX_TXIFRAMP"=181, "REG_IRQ_STATUS1_P2"=182, "REG_IRQ_STATUS2_P2"=183, "REG_IRQ_AUXSTATUS_P2"=184, "REG_MAC_UNLOCK"=188, "REG_MAC_TXIFFREQ"=190, "REG_WAKEUP_TESTCTRL1"=192, "REG_WAKEUP_RX_EN_CNT"=193, "REG_WAKEUP_TESTENABLES"=194, "REG_WAKEUP_DTBI_CTRL"=195, "REG_WAKEUP_DTBO_CTRL"=196, "REG_WAKEUP_TESTIOBUFTEST"=197, "REG_WAKEUP_WK_RX_TESTCTRL1"=198, "REG_WAKEUP_WK_RX_TESTCTRL2"=199, "REG_WAKEUP_SENS_SEQUENCE_CTRL"=200, "REG_WAKEUP_LNABIAS"=201, "REG_WAKEUP_DET_TH_TRIM1"=202, "REG_WAKEUP_LNABIAS_NOM1"=203, "REG_WAKEUP_RX_TSHORT_TRIM1"=204, "REG_WAKEUP_LNABIAS_NOM2"=205, "REG_WAKEUP_RX_TLONG_TRIM1"=206, "REG_WAKEUP_LNA_NEGRTRIM_NOM1"=207, "REG_WAKEUP_RX_TBURST_TRIM1"=208, "REG_WAKEUP_RX_LNA_NEGRTRIM_NOM2"=209, "REG_WAKEUP_RX_BB_G_BW_SEL1"=210, "REG_WAKEUP_WK_RX_DET_IOSTRIM1"=212, "REG_WAKEUP_WK_RX_CTRL2"=214, "REG_WAKEUP_WK_RX_RSSIVOSTRIM"=215, "REG_WAKEUP_LNANEGR_EFF"=216, "REG_WAKEUP_XOSU_FAST"=217, "REG_WAKEUP_STROSCPWIDTH1"=218, "REG_WAKEUP_STROSCPERIOD1"=220, "REG_WAKEUP_STROSCPERIOD2"=221, "REG_WAKEUP_WK_RX_LNA_NEGRTRIM1"=222, "REG_RF_TXTESTENABLE"=224, "REG_RF_TXIFTESTMODE"=225, "REG_RF_RXTESTENABLE"=226, "REG_RF_RXIFTESTCTRL1"=227, "REG_RF_RXIFTESTCTRL2"=228, "REG_RF_RXIFTESTCTRL3"=229, "REG_RF_SYNTH_TESTCTRL1"=230, "REG_RF_SYNTH_TESTCTRL2"=231, "REG_RF_SYNTH_TESTCTRL3"=232, "REG_RF_ADCTEST1"=237, "REG_RF_ADCTEST2"=238, "REG_RF_TXMIXER_IOSTRIM_LOW_IP"=240, "REG_RF_TXMIXER_IOSTRIM_LOW_IN"=241, "REG_RF_TXMIXER_ISOTRIM_LOW_QP"=242, "REG_RF_TXMIXER_IOSTRIM_LOW_QN"=243, "REG_RF_SYNTH_KPD"=244, "REG_RF_SYNTH_LOLEV"=245, "REG_RF_TXRFPWRTUNEANTSET"=246, "REG_RF_TXPD_GAIN_CTRL"=247, "REG_RF_SYNTH_STARTUP"=248, "REG_RF_TXRFANTTUNE_TXMODE"=249, "REG_RF_TXRFANTTUNE_RXMODE"=250, "REG_RF_RXRFANTTUNE_TXMODE"=251, "REG_RF_RXRFANTTUNE_RXMODE"=252, "REG_ANTMATCH1"=253, "REG_ANTMATCH2"=254, "REG_REVISION_P2"=255] ("Register")
      w33 = u16 74 items=["---MANUAL ENTRY---"=1000, "REG_NOREG"=0, "REG_RXBUFF_USED"=1, "REG_RXBUFF_BSIZE"=2, "REG_TXBUFF_USED"=3, "REG_TXBUFF_BSIZE"=4, "REG_TXBUFF_MAXPACKSIZE"=5, "REG_MAC_ERRCLR"=6, "REG_MAC_TRAINNUM"=7, "REG_MAC_SYNCMATCH"=8, "REG_MAC_SYNC1"=9, "REG_MAC_SYNC2"=10, "REG_MAC_SYNC3"=11, "REG_MAC_SYNC4"=12, "REG_MAC_SYNC5"=13, "REG_MAC_MAXBERR"=14, "REG_MAC_ECCORR"=15, "REG_MAC_CRCERR"=16, "REG_MAC_BLKCNT1"=17, "REG_MAC_BLKCNT2"=18, "REG_MAC_IMDTRANSID1"=19, "REG_MAC_IMDTRANSID2"=20, "REG_MAC_IMDTRANSID3"=21, "REG_MAC_COMPANYID"=22, "REG_MAC_MODUSER"=23, "REG_MAC_CHANNEL"=25, "REG_MAC_CLEARWDOG"=26, "REG_MAC_CKCORRTHRESH"=27, "REG_HK_TXADDR"=28, "REG_HK_TXDATA"=29, "REG_HK_TXREPLY"=30, "REG_HK_USERDATA"=31, "REG_HK_USERSTATUS"=32, "REG_HK_LASTADDRESS"=33, "REG_HK_MODE"=34, "REG_MAC_STATUSSEQ"=35, "REG_MAC_MAXRETRIES"=36, "REG_MAC_RESENDTIME"=37, "REG_MAC_POWERSAVETIME"=38, "REG_MAC_HEAD_DET"=39, "REG_MAC_CTRL"=41, "REG_MAC_INITCOM"=42, "REG_INTERFACE_MODE"=43, "REG_TXRXBUFF_BOTH"=44, "REG_TXRXBUFF"=45, "REG_IRQ_RAWSTATUS1"=46, "REG_IRQ_ENABLE1"=47, "REG_IRQ_ENABLESET1"=48, "REG_IRQ_ENABLECLEAR1"=49, "REG_IRQ_RAWSTATUS2"=50, "REG_IRQ_ENABLE2"=51, "REG_IRQ_ENABLESET2"=52, "REG_IRQ_ENABLECLEAR2"=53, "REG_IRQ_STATUS1"=54, "REG_IRQ_STATUS2"=55, "REG_IRQ_AUXSTATUS"=56, "REG_TXBUFF_OVERFLOW"=57, "REG_PO0"=58, "REG_P01"=59, "REG_P02"=60, "REG_P03"=61, "REG_GP0"=62, "REG_GPI"=63, "REG_WAKEUP_245IN"=64, "REG_WAKEUP_COMPANYID"=65, "REG_WAKEUP_IMDTRANSID1"=66, "REG_WAKEUP_IMDTRANSID2"=67, "REG_WAKEUP_IMDTRANSID3"=68, "REG_WAKEUP_CHANNEL"=69, "REG_WAKEUP_MODUSER"=70, "REG_WAKEUP_DEVICEMODE"=71, "REG_WAKEUP_WK_RX_CTRL1"=72, "REG_WAKEUP_STACK_ADDR"=73, "REG_WAKEUP_CTRL"=74, "REG_WAKEUP_STROSCRTRIM"=75, "REG_WAKEUP_BIASTRIM"=76, "REG_WAKEUP_ANT245TUNE"=77, "REG_WAKEUP_WK_RX_RTRIMDET"=78, "REG_WAKEUP_WK_RX_RTRIMDEMOD"=79, "REG_WAKEUP_WK_RX_RSSIGAIN"=80, "REG_WAKEUP_LNAFREQ1"=81, "REG_WAKEUP_STACK"=83, "REG_WAKUP_XOSU"=84, "REG_WAKUP_CNTDROPOUT"=85, "REG_WAKEUP_CRCCTRL"=86, "REG_WAKEUP_CRCWORD1"=87, "REG_WAKEUP_CRCWORD2"=88, "REG_WAKEUP_WK_RX_CTRIM"=89, "REG_WAKEUP_VDDATRIM"=90, "REG_WAKEUP_VDDDTRIM"=91, "REG_WAKEUP_TESTIOBUFEN"=92, "REG_WAKEUP_TESTIOCLAMP"=93, "CORE_RESET_ADDRESS"=94, "CHIP_RESET_ADDRESS"=95, "REG_RF_TXGENCTRL"=96, "REG_RF_TXIFCTRL"=97, "REG_RF_TXRF_SEL_CTRL"=98, "REG_RF_TXRFPWRDEFAULTSET"=99, "REG_RF_RSSITRIM"=100, "REG_RF_TXIFOSCTUNE"=101, "REG_RF_TXIFGAINIMB"=102, "REG_RF_TXIFLOCK"=103, "REG_RF_RXRFLNAGAINTRIM"=104, "REG_RF_RXBIASTR"=105, "REG_RF_RXGENCTRL"=106, "REG_RF_RXIFADCDECLEV"=107, "REG_RF_RXIFDETFILTERTUNE"=108, "REG_RF_RXIFFILTERTUNE"=109, "REG_RF_GENENABLES"=110, "REG_RF_SYNTH_CHANNEL"=111, "REG_TX_RAMP_RTRIM"=112, "REG_TX_RAMP_CTRIM"=113, "REG_RF_XO_TRIM"=114, "REG_RF_SYNTH_SET_TRIM"=115, "REG_RF_ADCCTRL"=116, "REG_RF_ADCOUTPUT"=117, "REG_RF_TXIFAMP"=118, "REG_RF_SYNTH_RTRIM"=119, "REG_RF_SYNTH_CTRIM"=120, "REG_RF_SYNTH_CT"=121, "REG_RF_TXMIXER_IOSTRIM_HIGH_IP"=122, "REG_RF_TXMIXER_IOSTRIM_HIGH_IN"=123, "REG_RF_TXMIXER_IOSTRIM_HIGH_QP"=124, "REG_RF_TXMIXER_IOSTRIM_HIGH_QN"=125, "REG_HX_WUADDR"=126, "REG_REVISION"=127, "REG_NOREG_TEST"=128, "REG_DTEST_RXBUFF"=129, "REG_RXBUFF_NEXT_BLOCK"=130, "REG_RXBUFF_FIRST_IN_PACK"=131, "REG_RXBUFF_FIRST_EMPTY"=132, "REG_MAC_BYPASS"=133, "REG_DTEST_TXBUFF"=134, "REG_TXBUFF_NEXT_BLOCK"=135, "REG_TXBUFF_FIRST_IN_PACK"=136, "REG_TXBUFF_FIRST_EMPTY"=137, "REG_DTEST_SEQ"=138, "REG_DTEST_CKCORR"=139, "REG_MAC_TOPSTATE"=140, "REG_DTEST_INTERFACE"=141, "REG_IFACE_TXRX_BYPASS"=142, "REG_MAC_TXRXWAIT"=143, "REG_MAC_TXRFRAMP"=144, "REG_MAC_TRAINWORD"=145, "REG_MAC_TRAINWORD2"=146, "REG_MAC_SETTINGS"=147, "REG_MAC_CALSELECT1"=148, "REG_MAC_CALSELECT2"=149, "REG_MAC_ANTMATCHSEL"=150, "REG_MAC_ANTTUNESEL1"=151, "REG_MAC_ANTTUNESEL2"=152, "REG_MAC_ANTTUNESEL3"=153, "REG_MAC_ANTTUNESTEP"=154, "REG_MAC_WUMODEBURST"=156, "REG_MAC_WUOFFSHORT"=157, "REG_MAC_WUOFFLONG"=158, "REG_MAC_CLKRECCTRL"=159, "REG_HK_MODE_P2"=162, "REG_MAC_ANTTUNERES1"=164, "REG_MAC_ANTTUNERES2"=165, "REG_INTERFACE_MODE_TEST"=171, "REG_TXRXBUFF_BOTH_P2"=172, "REG_TXRXBUFF_P2"=173, "REG_IRQ_RAWSTATUS1_P2"=174, "REG_MAC_TXIFSTATUS1"=176, "REG_MAC_TXIFSTATUS2"=177, "REG_IRQ_RAWSTATUS2_P2"=178, "REG_MAC_TXIFRAMPDELAY"=179, "REG_MAC_TXIFRAMPSLOPE"=180, "REG_MAX_TXIFRAMP"=181, "REG_IRQ_STATUS1_P2"=182, "REG_IRQ_STATUS2_P2"=183, "REG_IRQ_AUXSTATUS_P2"=184, "REG_MAC_UNLOCK"=188, "REG_MAC_TXIFFREQ"=190, "REG_WAKEUP_TESTCTRL1"=192, "REG_WAKEUP_RX_EN_CNT"=193, "REG_WAKEUP_TESTENABLES"=194, "REG_WAKEUP_DTBI_CTRL"=195, "REG_WAKEUP_DTBO_CTRL"=196, "REG_WAKEUP_TESTIOBUFTEST"=197, "REG_WAKEUP_WK_RX_TESTCTRL1"=198, "REG_WAKEUP_WK_RX_TESTCTRL2"=199, "REG_WAKEUP_SENS_SEQUENCE_CTRL"=200, "REG_WAKEUP_LNABIAS"=201, "REG_WAKEUP_DET_TH_TRIM1"=202, "REG_WAKEUP_LNABIAS_NOM1"=203, "REG_WAKEUP_RX_TSHORT_TRIM1"=204, "REG_WAKEUP_LNABIAS_NOM2"=205, "REG_WAKEUP_RX_TLONG_TRIM1"=206, "REG_WAKEUP_LNA_NEGRTRIM_NOM1"=207, "REG_WAKEUP_RX_TBURST_TRIM1"=208, "REG_WAKEUP_RX_LNA_NEGRTRIM_NOM2"=209, "REG_WAKEUP_RX_BB_G_BW_SEL1"=210, "REG_WAKEUP_WK_RX_DET_IOSTRIM1"=212, "REG_WAKEUP_WK_RX_CTRL2"=214, "REG_WAKEUP_WK_RX_RSSIVOSTRIM"=215, "REG_WAKEUP_LNANEGR_EFF"=216, "REG_WAKEUP_XOSU_FAST"=217, "REG_WAKEUP_STROSCPWIDTH1"=218, "REG_WAKEUP_STROSCPERIOD1"=220, "REG_WAKEUP_STROSCPERIOD2"=221, "REG_WAKEUP_WK_RX_LNA_NEGRTRIM1"=222, "REG_RF_TXTESTENABLE"=224, "REG_RF_TXIFTESTMODE"=225, "REG_RF_RXTESTENABLE"=226, "REG_RF_RXIFTESTCTRL1"=227, "REG_RF_RXIFTESTCTRL2"=228, "REG_RF_RXIFTESTCTRL3"=229, "REG_RF_SYNTH_TESTCTRL1"=230, "REG_RF_SYNTH_TESTCTRL2"=231, "REG_RF_SYNTH_TESTCTRL3"=232, "REG_RF_ADCTEST1"=237, "REG_RF_ADCTEST2"=238, "REG_RF_TXMIXER_IOSTRIM_LOW_IP"=240, "REG_RF_TXMIXER_IOSTRIM_LOW_IN"=241, "REG_RF_TXMIXER_ISOTRIM_LOW_QP"=242, "REG_RF_TXMIXER_IOSTRIM_LOW_QN"=243, "REG_RF_SYNTH_KPD"=244, "REG_RF_SYNTH_LOLEV"=245, "REG_RF_TXRFPWRTUNEANTSET"=246, "REG_RF_TXPD_GAIN_CTRL"=247, "REG_RF_SYNTH_STARTUP"=248, "REG_RF_TXRFANTTUNE_TXMODE"=249, "REG_RF_TXRFANTTUNE_RXMODE"=250, "REG_RF_RXRFANTTUNE_TXMODE"=251, "REG_RF_RXRFANTTUNE_RXMODE"=252, "REG_ANTMATCH1"=253, "REG_ANTMATCH2"=254, "REG_REVISION_P2"=255] ("Register")
      # "Enable RSSI, Wakeup LNA, Detector"
      # "Enable Wakeup Test Registers"
      # "Disable Wakeup Test Registers"
      n2 = call "MICSD Get Register.vi"("Execute on Remote?(F)"=w12, "error in (no error)"=w39, "Address"=w15, "VISA Resource Name"=w40) -> ("error out"=w20:errorcluster, "Data"=w18:u8, "dup VISA Resource Name"=w22:refnum<visa-resource-name>)  [unwired: 5 in]
      n3 = Or(x=u8 64 ("Data"), y=w18) -> (x .or. y?=w17:u8)
      n4 = call "MICSD Set Register.vi"("Execute on Remote?(F)"=w12, "error in (no error)"=w20, "Data"=w17, "Address"=w15, "VISA Resource Name"=w22) -> ("error out"=w19:errorcluster, "dup VISA Resource Name"=w21:refnum<visa-resource-name>)  [unwired: 5 in]
      n5 = call "MICSD Set Register.vi"("Execute on Remote?(F)"=w12, "error in (no error)"=w19, "Data"=u8 1, "Address"=w28, "VISA Resource Name"=w21) -> ("error out"=w23:errorcluster, "dup VISA Resource Name"=w24:refnum<visa-resource-name>)  [unwired: 5 in]
      n6 = call "MICSD Set Register.vi"("Execute on Remote?(F)"=w12, "error in (no error)"=w23, "Data"=u8 15, "Address"=w26, "VISA Resource Name"=w24) -> ("error out"=w30:errorcluster, "dup VISA Resource Name"=w29:refnum<visa-resource-name>)  [unwired: 5 in]
      n7 = case shown="\"Average, 20 Rdngs\"" w11 {
        tunnel: w29 -> [w55 w68]
        tunnel: w30 -> [w54 w67]
        tunnel: [w45 w66] -> w32
        tunnel: w12 -> [w42 w65]
        tunnel: [w44 w64] -> w31
        tunnel: w9 -> [_ w61]
        tunnel: [w42 w60] -> w10
        tunnel: [w41 w59] -> w8
        frame "Single Reading", Default {
          w47 = u16 117 items=["---MANUAL ENTRY---"=1000, "REG_NOREG"=0, "REG_RXBUFF_USED"=1, "REG_RXBUFF_BSIZE"=2, "REG_TXBUFF_USED"=3, "REG_TXBUFF_BSIZE"=4, "REG_TXBUFF_MAXPACKSIZE"=5, "REG_MAC_ERRCLR"=6, "REG_MAC_TRAINNUM"=7, "REG_MAC_SYNCMATCH"=8, "REG_MAC_SYNC1"=9, "REG_MAC_SYNC2"=10, "REG_MAC_SYNC3"=11, "REG_MAC_SYNC4"=12, "REG_MAC_SYNC5"=13, "REG_MAC_MAXBERR"=14, "REG_MAC_ECCORR"=15, "REG_MAC_CRCERR"=16, "REG_MAC_BLKCNT1"=17, "REG_MAC_BLKCNT2"=18, "REG_MAC_IMDTRANSID1"=19, "REG_MAC_IMDTRANSID2"=20, "REG_MAC_IMDTRANSID3"=21, "REG_MAC_COMPANYID"=22, "REG_MAC_MODUSER"=23, "REG_MAC_CHANNEL"=25, "REG_MAC_CLEARWDOG"=26, "REG_MAC_CKCORRTHRESH"=27, "REG_HK_TXADDR"=28, "REG_HK_TXDATA"=29, "REG_HK_TXREPLY"=30, "REG_HK_USERDATA"=31, "REG_HK_USERSTATUS"=32, "REG_HK_LASTADDRESS"=33, "REG_HK_MODE"=34, "REG_MAC_STATUSSEQ"=35, "REG_MAC_MAXRETRIES"=36, "REG_MAC_RESENDTIME"=37, "REG_MAC_POWERSAVETIME"=38, "REG_MAC_HEAD_DET"=39, "REG_MAC_CTRL"=41, "REG_MAC_INITCOM"=42, "REG_INTERFACE_MODE"=43, "REG_TXRXBUFF_BOTH"=44, "REG_TXRXBUFF"=45, "REG_IRQ_RAWSTATUS1"=46, "REG_IRQ_ENABLE1"=47, "REG_IRQ_ENABLESET1"=48, "REG_IRQ_ENABLECLEAR1"=49, "REG_IRQ_RAWSTATUS2"=50, "REG_IRQ_ENABLE2"=51, "REG_IRQ_ENABLESET2"=52, "REG_IRQ_ENABLECLEAR2"=53, "REG_IRQ_STATUS1"=54, "REG_IRQ_STATUS2"=55, "REG_IRQ_AUXSTATUS"=56, "REG_TXBUFF_OVERFLOW"=57, "REG_PO0"=58, "REG_P01"=59, "REG_P02"=60, "REG_P03"=61, "REG_GP0"=62, "REG_GPI"=63, "REG_WAKEUP_245IN"=64, "REG_WAKEUP_COMPANYID"=65, "REG_WAKEUP_IMDTRANSID1"=66, "REG_WAKEUP_IMDTRANSID2"=67, "REG_WAKEUP_IMDTRANSID3"=68, "REG_WAKEUP_CHANNEL"=69, "REG_WAKEUP_MODUSER"=70, "REG_WAKEUP_DEVICEMODE"=71, "REG_WAKEUP_WK_RX_CTRL1"=72, "REG_WAKEUP_STACK_ADDR"=73, "REG_WAKEUP_CTRL"=74, "REG_WAKEUP_STROSCRTRIM"=75, "REG_WAKEUP_BIASTRIM"=76, "REG_WAKEUP_ANT245TUNE"=77, "REG_WAKEUP_WK_RX_RTRIMDET"=78, "REG_WAKEUP_WK_RX_RTRIMDEMOD"=79, "REG_WAKEUP_WK_RX_RSSIGAIN"=80, "REG_WAKEUP_LNAFREQ1"=81, "REG_WAKEUP_STACK"=83, "REG_WAKUP_XOSU"=84, "REG_WAKUP_CNTDROPOUT"=85, "REG_WAKEUP_CRCCTRL"=86, "REG_WAKEUP_CRCWORD1"=87, "REG_WAKEUP_CRCWORD2"=88, "REG_WAKEUP_WK_RX_CTRIM"=89, "REG_WAKEUP_VDDATRIM"=90, "REG_WAKEUP_VDDDTRIM"=91, "REG_WAKEUP_TESTIOBUFEN"=92, "REG_WAKEUP_TESTIOCLAMP"=93, "CORE_RESET_ADDRESS"=94, "CHIP_RESET_ADDRESS"=95, "REG_RF_TXGENCTRL"=96, "REG_RF_TXIFCTRL"=97, "REG_RF_TXRF_SEL_CTRL"=98, "REG_RF_TXRFPWRDEFAULTSET"=99, "REG_RF_RSSITRIM"=100, "REG_RF_TXIFOSCTUNE"=101, "REG_RF_TXIFGAINIMB"=102, "REG_RF_TXIFLOCK"=103, "REG_RF_RXRFLNAGAINTRIM"=104, "REG_RF_RXBIASTR"=105, "REG_RF_RXGENCTRL"=106, "REG_RF_RXIFADCDECLEV"=107, "REG_RF_RXIFDETFILTERTUNE"=108, "REG_RF_RXIFFILTERTUNE"=109, "REG_RF_GENENABLES"=110, "REG_RF_SYNTH_CHANNEL"=111, "REG_TX_RAMP_RTRIM"=112, "REG_TX_RAMP_CTRIM"=113, "REG_RF_XO_TRIM"=114, "REG_RF_SYNTH_SET_TRIM"=115, "REG_RF_ADCCTRL"=116, "REG_RF_ADCOUTPUT"=117, "REG_RF_TXIFAMP"=118, "REG_RF_SYNTH_RTRIM"=119, "REG_RF_SYNTH_CTRIM"=120, "REG_RF_SYNTH_CT"=121, "REG_RF_TXMIXER_IOSTRIM_HIGH_IP"=122, "REG_RF_TXMIXER_IOSTRIM_HIGH_IN"=123, "REG_RF_TXMIXER_IOSTRIM_HIGH_QP"=124, "REG_RF_TXMIXER_IOSTRIM_HIGH_QN"=125, "REG_HX_WUADDR"=126, "REG_REVISION"=127, "REG_NOREG_TEST"=128, "REG_DTEST_RXBUFF"=129, "REG_RXBUFF_NEXT_BLOCK"=130, "REG_RXBUFF_FIRST_IN_PACK"=131, "REG_RXBUFF_FIRST_EMPTY"=132, "REG_MAC_BYPASS"=133, "REG_DTEST_TXBUFF"=134, "REG_TXBUFF_NEXT_BLOCK"=135, "REG_TXBUFF_FIRST_IN_PACK"=136, "REG_TXBUFF_FIRST_EMPTY"=137, "REG_DTEST_SEQ"=138, "REG_DTEST_CKCORR"=139, "REG_MAC_TOPSTATE"=140, "REG_DTEST_INTERFACE"=141, "REG_IFACE_TXRX_BYPASS"=142, "REG_MAC_TXRXWAIT"=143, "REG_MAC_TXRFRAMP"=144, "REG_MAC_TRAINWORD"=145, "REG_MAC_TRAINWORD2"=146, "REG_MAC_SETTINGS"=147, "REG_MAC_CALSELECT1"=148, "REG_MAC_CALSELECT2"=149, "REG_MAC_ANTMATCHSEL"=150, "REG_MAC_ANTTUNESEL1"=151, "REG_MAC_ANTTUNESEL2"=152, "REG_MAC_ANTTUNESEL3"=153, "REG_MAC_ANTTUNESTEP"=154, "REG_MAC_WUMODEBURST"=156, "REG_MAC_WUOFFSHORT"=157, "REG_MAC_WUOFFLONG"=158, "REG_MAC_CLKRECCTRL"=159, "REG_HK_MODE_P2"=162, "REG_MAC_ANTTUNERES1"=164, "REG_MAC_ANTTUNERES2"=165, "REG_INTERFACE_MODE_TEST"=171, "REG_TXRXBUFF_BOTH_P2"=172, "REG_TXRXBUFF_P2"=173, "REG_IRQ_RAWSTATUS1_P2"=174, "REG_MAC_TXIFSTATUS1"=176, "REG_MAC_TXIFSTATUS2"=177, "REG_IRQ_RAWSTATUS2_P2"=178, "REG_MAC_TXIFRAMPDELAY"=179, "REG_MAC_TXIFRAMPSLOPE"=180, "REG_MAX_TXIFRAMP"=181, "REG_IRQ_STATUS1_P2"=182, "REG_IRQ_STATUS2_P2"=183, "REG_IRQ_AUXSTATUS_P2"=184, "REG_MAC_UNLOCK"=188, "REG_MAC_TXIFFREQ"=190, "REG_WAKEUP_TESTCTRL1"=192, "REG_WAKEUP_RX_EN_CNT"=193, "REG_WAKEUP_TESTENABLES"=194, "REG_WAKEUP_DTBI_CTRL"=195, "REG_WAKEUP_DTBO_CTRL"=196, "REG_WAKEUP_TESTIOBUFTEST"=197, "REG_WAKEUP_WK_RX_TESTCTRL1"=198, "REG_WAKEUP_WK_RX_TESTCTRL2"=199, "REG_WAKEUP_SENS_SEQUENCE_CTRL"=200, "REG_WAKEUP_LNABIAS"=201, "REG_WAKEUP_DET_TH_TRIM1"=202, "REG_WAKEUP_LNABIAS_NOM1"=203, "REG_WAKEUP_RX_TSHORT_TRIM1"=204, "REG_WAKEUP_LNABIAS_NOM2"=205, "REG_WAKEUP_RX_TLONG_TRIM1"=206, "REG_WAKEUP_LNA_NEGRTRIM_NOM1"=207, "REG_WAKEUP_RX_TBURST_TRIM1"=208, "REG_WAKEUP_RX_LNA_NEGRTRIM_NOM2"=209, "REG_WAKEUP_RX_BB_G_BW_SEL1"=210, "REG_WAKEUP_WK_RX_DET_IOSTRIM1"=212, "REG_WAKEUP_WK_RX_CTRL2"=214, "REG_WAKEUP_WK_RX_RSSIVOSTRIM"=215, "REG_WAKEUP_LNANEGR_EFF"=216, "REG_WAKEUP_XOSU_FAST"=217, "REG_WAKEUP_STROSCPWIDTH1"=218, "REG_WAKEUP_STROSCPERIOD1"=220, "REG_WAKEUP_STROSCPERIOD2"=221, "REG_WAKEUP_WK_RX_LNA_NEGRTRIM1"=222, "REG_RF_TXTESTENABLE"=224, "REG_RF_TXIFTESTMODE"=225, "REG_RF_RXTESTENABLE"=226, "REG_RF_RXIFTESTCTRL1"=227, "REG_RF_RXIFTESTCTRL2"=228, "REG_RF_RXIFTESTCTRL3"=229, "REG_RF_SYNTH_TESTCTRL1"=230, "REG_RF_SYNTH_TESTCTRL2"=231, "REG_RF_SYNTH_TESTCTRL3"=232, "REG_RF_ADCTEST1"=237, "REG_RF_ADCTEST2"=238, "REG_RF_TXMIXER_IOSTRIM_LOW_IP"=240, "REG_RF_TXMIXER_IOSTRIM_LOW_IN"=241, "REG_RF_TXMIXER_ISOTRIM_LOW_QP"=242, "REG_RF_TXMIXER_IOSTRIM_LOW_QN"=243, "REG_RF_SYNTH_KPD"=244, "REG_RF_SYNTH_LOLEV"=245, "REG_RF_TXRFPWRTUNEANTSET"=246, "REG_RF_TXPD_GAIN_CTRL"=247, "REG_RF_SYNTH_STARTUP"=248, "REG_RF_TXRFANTTUNE_TXMODE"=249, "REG_RF_TXRFANTTUNE_RXMODE"=250, "REG_RF_RXRFANTTUNE_TXMODE"=251, "REG_RF_RXRFANTTUNE_RXMODE"=252, "REG_ANTMATCH1"=253, "REG_ANTMATCH2"=254, "REG_REVISION_P2"=255] ("Register")
          w52 = u16 116 items=["---MANUAL ENTRY---"=1000, "REG_NOREG"=0, "REG_RXBUFF_USED"=1, "REG_RXBUFF_BSIZE"=2, "REG_TXBUFF_USED"=3, "REG_TXBUFF_BSIZE"=4, "REG_TXBUFF_MAXPACKSIZE"=5, "REG_MAC_ERRCLR"=6, "REG_MAC_TRAINNUM"=7, "REG_MAC_SYNCMATCH"=8, "REG_MAC_SYNC1"=9, "REG_MAC_SYNC2"=10, "REG_MAC_SYNC3"=11, "REG_MAC_SYNC4"=12, "REG_MAC_SYNC5"=13, "REG_MAC_MAXBERR"=14, "REG_MAC_ECCORR"=15, "REG_MAC_CRCERR"=16, "REG_MAC_BLKCNT1"=17, "REG_MAC_BLKCNT2"=18, "REG_MAC_IMDTRANSID1"=19, "REG_MAC_IMDTRANSID2"=20, "REG_MAC_IMDTRANSID3"=21, "REG_MAC_COMPANYID"=22, "REG_MAC_MODUSER"=23, "REG_MAC_CHANNEL"=25, "REG_MAC_CLEARWDOG"=26, "REG_MAC_CKCORRTHRESH"=27, "REG_HK_TXADDR"=28, "REG_HK_TXDATA"=29, "REG_HK_TXREPLY"=30, "REG_HK_USERDATA"=31, "REG_HK_USERSTATUS"=32, "REG_HK_LASTADDRESS"=33, "REG_HK_MODE"=34, "REG_MAC_STATUSSEQ"=35, "REG_MAC_MAXRETRIES"=36, "REG_MAC_RESENDTIME"=37, "REG_MAC_POWERSAVETIME"=38, "REG_MAC_HEAD_DET"=39, "REG_MAC_CTRL"=41, "REG_MAC_INITCOM"=42, "REG_INTERFACE_MODE"=43, "REG_TXRXBUFF_BOTH"=44, "REG_TXRXBUFF"=45, "REG_IRQ_RAWSTATUS1"=46, "REG_IRQ_ENABLE1"=47, "REG_IRQ_ENABLESET1"=48, "REG_IRQ_ENABLECLEAR1"=49, "REG_IRQ_RAWSTATUS2"=50, "REG_IRQ_ENABLE2"=51, "REG_IRQ_ENABLESET2"=52, "REG_IRQ_ENABLECLEAR2"=53, "REG_IRQ_STATUS1"=54, "REG_IRQ_STATUS2"=55, "REG_IRQ_AUXSTATUS"=56, "REG_TXBUFF_OVERFLOW"=57, "REG_PO0"=58, "REG_P01"=59, "REG_P02"=60, "REG_P03"=61, "REG_GP0"=62, "REG_GPI"=63, "REG_WAKEUP_245IN"=64, "REG_WAKEUP_COMPANYID"=65, "REG_WAKEUP_IMDTRANSID1"=66, "REG_WAKEUP_IMDTRANSID2"=67, "REG_WAKEUP_IMDTRANSID3"=68, "REG_WAKEUP_CHANNEL"=69, "REG_WAKEUP_MODUSER"=70, "REG_WAKEUP_DEVICEMODE"=71, "REG_WAKEUP_WK_RX_CTRL1"=72, "REG_WAKEUP_STACK_ADDR"=73, "REG_WAKEUP_CTRL"=74, "REG_WAKEUP_STROSCRTRIM"=75, "REG_WAKEUP_BIASTRIM"=76, "REG_WAKEUP_ANT245TUNE"=77, "REG_WAKEUP_WK_RX_RTRIMDET"=78, "REG_WAKEUP_WK_RX_RTRIMDEMOD"=79, "REG_WAKEUP_WK_RX_RSSIGAIN"=80, "REG_WAKEUP_LNAFREQ1"=81, "REG_WAKEUP_STACK"=83, "REG_WAKUP_XOSU"=84, "REG_WAKUP_CNTDROPOUT"=85, "REG_WAKEUP_CRCCTRL"=86, "REG_WAKEUP_CRCWORD1"=87, "REG_WAKEUP_CRCWORD2"=88, "REG_WAKEUP_WK_RX_CTRIM"=89, "REG_WAKEUP_VDDATRIM"=90, "REG_WAKEUP_VDDDTRIM"=91, "REG_WAKEUP_TESTIOBUFEN"=92, "REG_WAKEUP_TESTIOCLAMP"=93, "CORE_RESET_ADDRESS"=94, "CHIP_RESET_ADDRESS"=95, "REG_RF_TXGENCTRL"=96, "REG_RF_TXIFCTRL"=97, "REG_RF_TXRF_SEL_CTRL"=98, "REG_RF_TXRFPWRDEFAULTSET"=99, "REG_RF_RSSITRIM"=100, "REG_RF_TXIFOSCTUNE"=101, "REG_RF_TXIFGAINIMB"=102, "REG_RF_TXIFLOCK"=103, "REG_RF_RXRFLNAGAINTRIM"=104, "REG_RF_RXBIASTR"=105, "REG_RF_RXGENCTRL"=106, "REG_RF_RXIFADCDECLEV"=107, "REG_RF_RXIFDETFILTERTUNE"=108, "REG_RF_RXIFFILTERTUNE"=109, "REG_RF_GENENABLES"=110, "REG_RF_SYNTH_CHANNEL"=111, "REG_TX_RAMP_RTRIM"=112, "REG_TX_RAMP_CTRIM"=113, "REG_RF_XO_TRIM"=114, "REG_RF_SYNTH_SET_TRIM"=115, "REG_RF_ADCCTRL"=116, "REG_RF_ADCOUTPUT"=117, "REG_RF_TXIFAMP"=118, "REG_RF_SYNTH_RTRIM"=119, "REG_RF_SYNTH_CTRIM"=120, "REG_RF_SYNTH_CT"=121, "REG_RF_TXMIXER_IOSTRIM_HIGH_IP"=122, "REG_RF_TXMIXER_IOSTRIM_HIGH_IN"=123, "REG_RF_TXMIXER_IOSTRIM_HIGH_QP"=124, "REG_RF_TXMIXER_IOSTRIM_HIGH_QN"=125, "REG_HX_WUADDR"=126, "REG_REVISION"=127, "REG_NOREG_TEST"=128, "REG_DTEST_RXBUFF"=129, "REG_RXBUFF_NEXT_BLOCK"=130, "REG_RXBUFF_FIRST_IN_PACK"=131, "REG_RXBUFF_FIRST_EMPTY"=132, "REG_MAC_BYPASS"=133, "REG_DTEST_TXBUFF"=134, "REG_TXBUFF_NEXT_BLOCK"=135, "REG_TXBUFF_FIRST_IN_PACK"=136, "REG_TXBUFF_FIRST_EMPTY"=137, "REG_DTEST_SEQ"=138, "REG_DTEST_CKCORR"=139, "REG_MAC_TOPSTATE"=140, "REG_DTEST_INTERFACE"=141, "REG_IFACE_TXRX_BYPASS"=142, "REG_MAC_TXRXWAIT"=143, "REG_MAC_TXRFRAMP"=144, "REG_MAC_TRAINWORD"=145, "REG_MAC_TRAINWORD2"=146, "REG_MAC_SETTINGS"=147, "REG_MAC_CALSELECT1"=148, "REG_MAC_CALSELECT2"=149, "REG_MAC_ANTMATCHSEL"=150, "REG_MAC_ANTTUNESEL1"=151, "REG_MAC_ANTTUNESEL2"=152, "REG_MAC_ANTTUNESEL3"=153, "REG_MAC_ANTTUNESTEP"=154, "REG_MAC_WUMODEBURST"=156, "REG_MAC_WUOFFSHORT"=157, "REG_MAC_WUOFFLONG"=158, "REG_MAC_CLKRECCTRL"=159, "REG_HK_MODE_P2"=162, "REG_MAC_ANTTUNERES1"=164, "REG_MAC_ANTTUNERES2"=165, "REG_INTERFACE_MODE_TEST"=171, "REG_TXRXBUFF_BOTH_P2"=172, "REG_TXRXBUFF_P2"=173, "REG_IRQ_RAWSTATUS1_P2"=174, "REG_MAC_TXIFSTATUS1"=176, "REG_MAC_TXIFSTATUS2"=177, "REG_IRQ_RAWSTATUS2_P2"=178, "REG_MAC_TXIFRAMPDELAY"=179, "REG_MAC_TXIFRAMPSLOPE"=180, "REG_MAX_TXIFRAMP"=181, "REG_IRQ_STATUS1_P2"=182, "REG_IRQ_STATUS2_P2"=183, "REG_IRQ_AUXSTATUS_P2"=184, "REG_MAC_UNLOCK"=188, "REG_MAC_TXIFFREQ"=190, "REG_WAKEUP_TESTCTRL1"=192, "REG_WAKEUP_RX_EN_CNT"=193, "REG_WAKEUP_TESTENABLES"=194, "REG_WAKEUP_DTBI_CTRL"=195, "REG_WAKEUP_DTBO_CTRL"=196, "REG_WAKEUP_TESTIOBUFTEST"=197, "REG_WAKEUP_WK_RX_TESTCTRL1"=198, "REG_WAKEUP_WK_RX_TESTCTRL2"=199, "REG_WAKEUP_SENS_SEQUENCE_CTRL"=200, "REG_WAKEUP_LNABIAS"=201, "REG_WAKEUP_DET_TH_TRIM1"=202, "REG_WAKEUP_LNABIAS_NOM1"=203, "REG_WAKEUP_RX_TSHORT_TRIM1"=204, "REG_WAKEUP_LNABIAS_NOM2"=205, "REG_WAKEUP_RX_TLONG_TRIM1"=206, "REG_WAKEUP_LNA_NEGRTRIM_NOM1"=207, "REG_WAKEUP_RX_TBURST_TRIM1"=208, "REG_WAKEUP_RX_LNA_NEGRTRIM_NOM2"=209, "REG_WAKEUP_RX_BB_G_BW_SEL1"=210, "REG_WAKEUP_WK_RX_DET_IOSTRIM1"=212, "REG_WAKEUP_WK_RX_CTRL2"=214, "REG_WAKEUP_WK_RX_RSSIVOSTRIM"=215, "REG_WAKEUP_LNANEGR_EFF"=216, "REG_WAKEUP_XOSU_FAST"=217, "REG_WAKEUP_STROSCPWIDTH1"=218, "REG_WAKEUP_STROSCPERIOD1"=220, "REG_WAKEUP_STROSCPERIOD2"=221, "REG_WAKEUP_WK_RX_LNA_NEGRTRIM1"=222, "REG_RF_TXTESTENABLE"=224, "REG_RF_TXIFTESTMODE"=225, "REG_RF_RXTESTENABLE"=226, "REG_RF_RXIFTESTCTRL1"=227, "REG_RF_RXIFTESTCTRL2"=228, "REG_RF_RXIFTESTCTRL3"=229, "REG_RF_SYNTH_TESTCTRL1"=230, "REG_RF_SYNTH_TESTCTRL2"=231, "REG_RF_SYNTH_TESTCTRL3"=232, "REG_RF_ADCTEST1"=237, "REG_RF_ADCTEST2"=238, "REG_RF_TXMIXER_IOSTRIM_LOW_IP"=240, "REG_RF_TXMIXER_IOSTRIM_LOW_IN"=241, "REG_RF_TXMIXER_ISOTRIM_LOW_QP"=242, "REG_RF_TXMIXER_IOSTRIM_LOW_QN"=243, "REG_RF_SYNTH_KPD"=244, "REG_RF_SYNTH_LOLEV"=245, "REG_RF_TXRFPWRTUNEANTSET"=246, "REG_RF_TXPD_GAIN_CTRL"=247, "REG_RF_SYNTH_STARTUP"=248, "REG_RF_TXRFANTTUNE_TXMODE"=249, "REG_RF_TXRFANTTUNE_RXMODE"=250, "REG_RF_RXRFANTTUNE_TXMODE"=251, "REG_RF_RXRFANTTUNE_RXMODE"=252, "REG_ANTMATCH1"=253, "REG_ANTMATCH2"=254, "REG_REVISION_P2"=255] ("Register")
          n8 = call "MICSD Set Register.vi"("Execute on Remote?(F)"=w42, "error in (no error)"=w54, "Data"=u8 29, "Address"=w52, "VISA Resource Name"=w55) -> ("error out"=w56:errorcluster, "dup VISA Resource Name"=w57:refnum<visa-resource-name>)  [unwired: 5 in]
          n9 = call "MICSD Set Register.vi"("Execute on Remote?(F)"=w42, "error in (no error)"=w56, "Data"=u8 31, "Address"=w52, "VISA Resource Name"=w57) -> ("error out"=w51:errorcluster, "dup VISA Resource Name"=w48:refnum<visa-resource-name>)  [unwired: 5 in]
          n10 = call "Simple Wait.vi"("mS"=u32 20, "error in"=w51) -> ("error out"=w49:errorcluster)  [unwired: 12 in, 1 out]
          n11 = call "MICSD Get Register.vi"("Execute on Remote?(F)"=w42, "error in (no error)"=w49, "Address"=w47, "VISA Resource Name"=w48) -> ("error out"=w45:errorcluster, "Data"=w46:u8, "dup VISA Resource Name"=w44:refnum<visa-resource-name>)  [unwired: 5 in]
          n12 = Subtract(x=w46, y=u8 32) -> (x-y=w41:u8)
        }
        frame "Average, 20 Rdngs" {
          n13 = for {
            N: w61 -> [_]
            tunnel: w68 -> [w84]
            tunnel: w65 -> [w69]
            tunnel: [w73] -> w64
            tunnel: [w72] -> w63 mode=indexing
            shift-right: [w74] -> w66
            shift-left: w67 -> [w83]
            tunnel: [w69] -> w60
            w76 = u16 117 items=["---MANUAL ENTRY---"=1000, "REG_NOREG"=0, "REG_RXBUFF_USED"=1, "REG_RXBUFF_BSIZE"=2, "REG_TXBUFF_USED"=3, "REG_TXBUFF_BSIZE"=4, "REG_TXBUFF_MAXPACKSIZE"=5, "REG_MAC_ERRCLR"=6, "REG_MAC_TRAINNUM"=7, "REG_MAC_SYNCMATCH"=8, "REG_MAC_SYNC1"=9, "REG_MAC_SYNC2"=10, "REG_MAC_SYNC3"=11, "REG_MAC_SYNC4"=12, "REG_MAC_SYNC5"=13, "REG_MAC_MAXBERR"=14, "REG_MAC_ECCORR"=15, "REG_MAC_CRCERR"=16, "REG_MAC_BLKCNT1"=17, "REG_MAC_BLKCNT2"=18, "REG_MAC_IMDTRANSID1"=19, "REG_MAC_IMDTRANSID2"=20, "REG_MAC_IMDTRANSID3"=21, "REG_MAC_COMPANYID"=22, "REG_MAC_MODUSER"=23, "REG_MAC_CHANNEL"=25, "REG_MAC_CLEARWDOG"=26, "REG_MAC_CKCORRTHRESH"=27, "REG_HK_TXADDR"=28, "REG_HK_TXDATA"=29, "REG_HK_TXREPLY"=30, "REG_HK_USERDATA"=31, "REG_HK_USERSTATUS"=32, "REG_HK_LASTADDRESS"=33, "REG_HK_MODE"=34, "REG_MAC_STATUSSEQ"=35, "REG_MAC_MAXRETRIES"=36, "REG_MAC_RESENDTIME"=37, "REG_MAC_POWERSAVETIME"=38, "REG_MAC_HEAD_DET"=39, "REG_MAC_CTRL"=41, "REG_MAC_INITCOM"=42, "REG_INTERFACE_MODE"=43, "REG_TXRXBUFF_BOTH"=44, "REG_TXRXBUFF"=45, "REG_IRQ_RAWSTATUS1"=46, "REG_IRQ_ENABLE1"=47, "REG_IRQ_ENABLESET1"=48, "REG_IRQ_ENABLECLEAR1"=49, "REG_IRQ_RAWSTATUS2"=50, "REG_IRQ_ENABLE2"=51, "REG_IRQ_ENABLESET2"=52, "REG_IRQ_ENABLECLEAR2"=53, "REG_IRQ_STATUS1"=54, "REG_IRQ_STATUS2"=55, "REG_IRQ_AUXSTATUS"=56, "REG_TXBUFF_OVERFLOW"=57, "REG_PO0"=58, "REG_P01"=59, "REG_P02"=60, "REG_P03"=61, "REG_GP0"=62, "REG_GPI"=63, "REG_WAKEUP_245IN"=64, "REG_WAKEUP_COMPANYID"=65, "REG_WAKEUP_IMDTRANSID1"=66, "REG_WAKEUP_IMDTRANSID2"=67, "REG_WAKEUP_IMDTRANSID3"=68, "REG_WAKEUP_CHANNEL"=69, "REG_WAKEUP_MODUSER"=70, "REG_WAKEUP_DEVICEMODE"=71, "REG_WAKEUP_WK_RX_CTRL1"=72, "REG_WAKEUP_STACK_ADDR"=73, "REG_WAKEUP_CTRL"=74, "REG_WAKEUP_STROSCRTRIM"=75, "REG_WAKEUP_BIASTRIM"=76, "REG_WAKEUP_ANT245TUNE"=77, "REG_WAKEUP_WK_RX_RTRIMDET"=78, "REG_WAKEUP_WK_RX_RTRIMDEMOD"=79, "REG_WAKEUP_WK_RX_RSSIGAIN"=80, "REG_WAKEUP_LNAFREQ1"=81, "REG_WAKEUP_STACK"=83, "REG_WAKUP_XOSU"=84, "REG_WAKUP_CNTDROPOUT"=85, "REG_WAKEUP_CRCCTRL"=86, "REG_WAKEUP_CRCWORD1"=87, "REG_WAKEUP_CRCWORD2"=88, "REG_WAKEUP_WK_RX_CTRIM"=89, "REG_WAKEUP_VDDATRIM"=90, "REG_WAKEUP_VDDDTRIM"=91, "REG_WAKEUP_TESTIOBUFEN"=92, "REG_WAKEUP_TESTIOCLAMP"=93, "CORE_RESET_ADDRESS"=94, "CHIP_RESET_ADDRESS"=95, "REG_RF_TXGENCTRL"=96, "REG_RF_TXIFCTRL"=97, "REG_RF_TXRF_SEL_CTRL"=98, "REG_RF_TXRFPWRDEFAULTSET"=99, "REG_RF_RSSITRIM"=100, "REG_RF_TXIFOSCTUNE"=101, "REG_RF_TXIFGAINIMB"=102, "REG_RF_TXIFLOCK"=103, "REG_RF_RXRFLNAGAINTRIM"=104, "REG_RF_RXBIASTR"=105, "REG_RF_RXGENCTRL"=106, "REG_RF_RXIFADCDECLEV"=107, "REG_RF_RXIFDETFILTERTUNE"=108, "REG_RF_RXIFFILTERTUNE"=109, "REG_RF_GENENABLES"=110, "REG_RF_SYNTH_CHANNEL"=111, "REG_TX_RAMP_RTRIM"=112, "REG_TX_RAMP_CTRIM"=113, "REG_RF_XO_TRIM"=114, "REG_RF_SYNTH_SET_TRIM"=115, "REG_RF_ADCCTRL"=116, "REG_RF_ADCOUTPUT"=117, "REG_RF_TXIFAMP"=118, "REG_RF_SYNTH_RTRIM"=119, "REG_RF_SYNTH_CTRIM"=120, "REG_RF_SYNTH_CT"=121, "REG_RF_TXMIXER_IOSTRIM_HIGH_IP"=122, "REG_RF_TXMIXER_IOSTRIM_HIGH_IN"=123, "REG_RF_TXMIXER_IOSTRIM_HIGH_QP"=124, "REG_RF_TXMIXER_IOSTRIM_HIGH_QN"=125, "REG_HX_WUADDR"=126, "REG_REVISION"=127, "REG_NOREG_TEST"=128, "REG_DTEST_RXBUFF"=129, "REG_RXBUFF_NEXT_BLOCK"=130, "REG_RXBUFF_FIRST_IN_PACK"=131, "REG_RXBUFF_FIRST_EMPTY"=132, "REG_MAC_BYPASS"=133, "REG_DTEST_TXBUFF"=134, "REG_TXBUFF_NEXT_BLOCK"=135, "REG_TXBUFF_FIRST_IN_PACK"=136, "REG_TXBUFF_FIRST_EMPTY"=137, "REG_DTEST_SEQ"=138, "REG_DTEST_CKCORR"=139, "REG_MAC_TOPSTATE"=140, "REG_DTEST_INTERFACE"=141, "REG_IFACE_TXRX_BYPASS"=142, "REG_MAC_TXRXWAIT"=143, "REG_MAC_TXRFRAMP"=144, "REG_MAC_TRAINWORD"=145, "REG_MAC_TRAINWORD2"=146, "REG_MAC_SETTINGS"=147, "REG_MAC_CALSELECT1"=148, "REG_MAC_CALSELECT2"=149, "REG_MAC_ANTMATCHSEL"=150, "REG_MAC_ANTTUNESEL1"=151, "REG_MAC_ANTTUNESEL2"=152, "REG_MAC_ANTTUNESEL3"=153, "REG_MAC_ANTTUNESTEP"=154, "REG_MAC_WUMODEBURST"=156, "REG_MAC_WUOFFSHORT"=157, "REG_MAC_WUOFFLONG"=158, "REG_MAC_CLKRECCTRL"=159, "REG_HK_MODE_P2"=162, "REG_MAC_ANTTUNERES1"=164, "REG_MAC_ANTTUNERES2"=165, "REG_INTERFACE_MODE_TEST"=171, "REG_TXRXBUFF_BOTH_P2"=172, "REG_TXRXBUFF_P2"=173, "REG_IRQ_RAWSTATUS1_P2"=174, "REG_MAC_TXIFSTATUS1"=176, "REG_MAC_TXIFSTATUS2"=177, "REG_IRQ_RAWSTATUS2_P2"=178, "REG_MAC_TXIFRAMPDELAY"=179, "REG_MAC_TXIFRAMPSLOPE"=180, "REG_MAX_TXIFRAMP"=181, "REG_IRQ_STATUS1_P2"=182, "REG_IRQ_STATUS2_P2"=183, "REG_IRQ_AUXSTATUS_P2"=184, "REG_MAC_UNLOCK"=188, "REG_MAC_TXIFFREQ"=190, "REG_WAKEUP_TESTCTRL1"=192, "REG_WAKEUP_RX_EN_CNT"=193, "REG_WAKEUP_TESTENABLES"=194, "REG_WAKEUP_DTBI_CTRL"=195, "REG_WAKEUP_DTBO_CTRL"=196, "REG_WAKEUP_TESTIOBUFTEST"=197, "REG_WAKEUP_WK_RX_TESTCTRL1"=198, "REG_WAKEUP_WK_RX_TESTCTRL2"=199, "REG_WAKEUP_SENS_SEQUENCE_CTRL"=200, "REG_WAKEUP_LNABIAS"=201, "REG_WAKEUP_DET_TH_TRIM1"=202, "REG_WAKEUP_LNABIAS_NOM1"=203, "REG_WAKEUP_RX_TSHORT_TRIM1"=204, "REG_WAKEUP_LNABIAS_NOM2"=205, "REG_WAKEUP_RX_TLONG_TRIM1"=206, "REG_WAKEUP_LNA_NEGRTRIM_NOM1"=207, "REG_WAKEUP_RX_TBURST_TRIM1"=208, "REG_WAKEUP_RX_LNA_NEGRTRIM_NOM2"=209, "REG_WAKEUP_RX_BB_G_BW_SEL1"=210, "REG_WAKEUP_WK_RX_DET_IOSTRIM1"=212, "REG_WAKEUP_WK_RX_CTRL2"=214, "REG_WAKEUP_WK_RX_RSSIVOSTRIM"=215, "REG_WAKEUP_LNANEGR_EFF"=216, "REG_WAKEUP_XOSU_FAST"=217, "REG_WAKEUP_STROSCPWIDTH1"=218, "REG_WAKEUP_STROSCPERIOD1"=220, "REG_WAKEUP_STROSCPERIOD2"=221, "REG_WAKEUP_WK_RX_LNA_NEGRTRIM1"=222, "REG_RF_TXTESTENABLE"=224, "REG_RF_TXIFTESTMODE"=225, "REG_RF_RXTESTENABLE"=226, "REG_RF_RXIFTESTCTRL1"=227, "REG_RF_RXIFTESTCTRL2"=228, "REG_RF_RXIFTESTCTRL3"=229, "REG_RF_SYNTH_TESTCTRL1"=230, "REG_RF_SYNTH_TESTCTRL2"=231, "REG_RF_SYNTH_TESTCTRL3"=232, "REG_RF_ADCTEST1"=237, "REG_RF_ADCTEST2"=238, "REG_RF_TXMIXER_IOSTRIM_LOW_IP"=240, "REG_RF_TXMIXER_IOSTRIM_LOW_IN"=241, "REG_RF_TXMIXER_ISOTRIM_LOW_QP"=242, "REG_RF_TXMIXER_IOSTRIM_LOW_QN"=243, "REG_RF_SYNTH_KPD"=244, "REG_RF_SYNTH_LOLEV"=245, "REG_RF_TXRFPWRTUNEANTSET"=246, "REG_RF_TXPD_GAIN_CTRL"=247, "REG_RF_SYNTH_STARTUP"=248, "REG_RF_TXRFANTTUNE_TXMODE"=249, "REG_RF_TXRFANTTUNE_RXMODE"=250, "REG_RF_RXRFANTTUNE_TXMODE"=251, "REG_RF_RXRFANTTUNE_RXMODE"=252, "REG_ANTMATCH1"=253, "REG_ANTMATCH2"=254, "REG_REVISION_P2"=255] ("Register")
            w81 = u16 116 items=["---MANUAL ENTRY---"=1000, "REG_NOREG"=0, "REG_RXBUFF_USED"=1, "REG_RXBUFF_BSIZE"=2, "REG_TXBUFF_USED"=3, "REG_TXBUFF_BSIZE"=4, "REG_TXBUFF_MAXPACKSIZE"=5, "REG_MAC_ERRCLR"=6, "REG_MAC_TRAINNUM"=7, "REG_MAC_SYNCMATCH"=8, "REG_MAC_SYNC1"=9, "REG_MAC_SYNC2"=10, "REG_MAC_SYNC3"=11, "REG_MAC_SYNC4"=12, "REG_MAC_SYNC5"=13, "REG_MAC_MAXBERR"=14, "REG_MAC_ECCORR"=15, "REG_MAC_CRCERR"=16, "REG_MAC_BLKCNT1"=17, "REG_MAC_BLKCNT2"=18, "REG_MAC_IMDTRANSID1"=19, "REG_MAC_IMDTRANSID2"=20, "REG_MAC_IMDTRANSID3"=21, "REG_MAC_COMPANYID"=22, "REG_MAC_MODUSER"=23, "REG_MAC_CHANNEL"=25, "REG_MAC_CLEARWDOG"=26, "REG_MAC_CKCORRTHRESH"=27, "REG_HK_TXADDR"=28, "REG_HK_TXDATA"=29, "REG_HK_TXREPLY"=30, "REG_HK_USERDATA"=31, "REG_HK_USERSTATUS"=32, "REG_HK_LASTADDRESS"=33, "REG_HK_MODE"=34, "REG_MAC_STATUSSEQ"=35, "REG_MAC_MAXRETRIES"=36, "REG_MAC_RESENDTIME"=37, "REG_MAC_POWERSAVETIME"=38, "REG_MAC_HEAD_DET"=39, "REG_MAC_CTRL"=41, "REG_MAC_INITCOM"=42, "REG_INTERFACE_MODE"=43, "REG_TXRXBUFF_BOTH"=44, "REG_TXRXBUFF"=45, "REG_IRQ_RAWSTATUS1"=46, "REG_IRQ_ENABLE1"=47, "REG_IRQ_ENABLESET1"=48, "REG_IRQ_ENABLECLEAR1"=49, "REG_IRQ_RAWSTATUS2"=50, "REG_IRQ_ENABLE2"=51, "REG_IRQ_ENABLESET2"=52, "REG_IRQ_ENABLECLEAR2"=53, "REG_IRQ_STATUS1"=54, "REG_IRQ_STATUS2"=55, "REG_IRQ_AUXSTATUS"=56, "REG_TXBUFF_OVERFLOW"=57, "REG_PO0"=58, "REG_P01"=59, "REG_P02"=60, "REG_P03"=61, "REG_GP0"=62, "REG_GPI"=63, "REG_WAKEUP_245IN"=64, "REG_WAKEUP_COMPANYID"=65, "REG_WAKEUP_IMDTRANSID1"=66, "REG_WAKEUP_IMDTRANSID2"=67, "REG_WAKEUP_IMDTRANSID3"=68, "REG_WAKEUP_CHANNEL"=69, "REG_WAKEUP_MODUSER"=70, "REG_WAKEUP_DEVICEMODE"=71, "REG_WAKEUP_WK_RX_CTRL1"=72, "REG_WAKEUP_STACK_ADDR"=73, "REG_WAKEUP_CTRL"=74, "REG_WAKEUP_STROSCRTRIM"=75, "REG_WAKEUP_BIASTRIM"=76, "REG_WAKEUP_ANT245TUNE"=77, "REG_WAKEUP_WK_RX_RTRIMDET"=78, "REG_WAKEUP_WK_RX_RTRIMDEMOD"=79, "REG_WAKEUP_WK_RX_RSSIGAIN"=80, "REG_WAKEUP_LNAFREQ1"=81, "REG_WAKEUP_STACK"=83, "REG_WAKUP_XOSU"=84, "REG_WAKUP_CNTDROPOUT"=85, "REG_WAKEUP_CRCCTRL"=86, "REG_WAKEUP_CRCWORD1"=87, "REG_WAKEUP_CRCWORD2"=88, "REG_WAKEUP_WK_RX_CTRIM"=89, "REG_WAKEUP_VDDATRIM"=90, "REG_WAKEUP_VDDDTRIM"=91, "REG_WAKEUP_TESTIOBUFEN"=92, "REG_WAKEUP_TESTIOCLAMP"=93, "CORE_RESET_ADDRESS"=94, "CHIP_RESET_ADDRESS"=95, "REG_RF_TXGENCTRL"=96, "REG_RF_TXIFCTRL"=97, "REG_RF_TXRF_SEL_CTRL"=98, "REG_RF_TXRFPWRDEFAULTSET"=99, "REG_RF_RSSITRIM"=100, "REG_RF_TXIFOSCTUNE"=101, "REG_RF_TXIFGAINIMB"=102, "REG_RF_TXIFLOCK"=103, "REG_RF_RXRFLNAGAINTRIM"=104, "REG_RF_RXBIASTR"=105, "REG_RF_RXGENCTRL"=106, "REG_RF_RXIFADCDECLEV"=107, "REG_RF_RXIFDETFILTERTUNE"=108, "REG_RF_RXIFFILTERTUNE"=109, "REG_RF_GENENABLES"=110, "REG_RF_SYNTH_CHANNEL"=111, "REG_TX_RAMP_RTRIM"=112, "REG_TX_RAMP_CTRIM"=113, "REG_RF_XO_TRIM"=114, "REG_RF_SYNTH_SET_TRIM"=115, "REG_RF_ADCCTRL"=116, "REG_RF_ADCOUTPUT"=117, "REG_RF_TXIFAMP"=118, "REG_RF_SYNTH_RTRIM"=119, "REG_RF_SYNTH_CTRIM"=120, "REG_RF_SYNTH_CT"=121, "REG_RF_TXMIXER_IOSTRIM_HIGH_IP"=122, "REG_RF_TXMIXER_IOSTRIM_HIGH_IN"=123, "REG_RF_TXMIXER_IOSTRIM_HIGH_QP"=124, "REG_RF_TXMIXER_IOSTRIM_HIGH_QN"=125, "REG_HX_WUADDR"=126, "REG_REVISION"=127, "REG_NOREG_TEST"=128, "REG_DTEST_RXBUFF"=129, "REG_RXBUFF_NEXT_BLOCK"=130, "REG_RXBUFF_FIRST_IN_PACK"=131, "REG_RXBUFF_FIRST_EMPTY"=132, "REG_MAC_BYPASS"=133, "REG_DTEST_TXBUFF"=134, "REG_TXBUFF_NEXT_BLOCK"=135, "REG_TXBUFF_FIRST_IN_PACK"=136, "REG_TXBUFF_FIRST_EMPTY"=137, "REG_DTEST_SEQ"=138, "REG_DTEST_CKCORR"=139, "REG_MAC_TOPSTATE"=140, "REG_DTEST_INTERFACE"=141, "REG_IFACE_TXRX_BYPASS"=142, "REG_MAC_TXRXWAIT"=143, "REG_MAC_TXRFRAMP"=144, "REG_MAC_TRAINWORD"=145, "REG_MAC_TRAINWORD2"=146, "REG_MAC_SETTINGS"=147, "REG_MAC_CALSELECT1"=148, "REG_MAC_CALSELECT2"=149, "REG_MAC_ANTMATCHSEL"=150, "REG_MAC_ANTTUNESEL1"=151, "REG_MAC_ANTTUNESEL2"=152, "REG_MAC_ANTTUNESEL3"=153, "REG_MAC_ANTTUNESTEP"=154, "REG_MAC_WUMODEBURST"=156, "REG_MAC_WUOFFSHORT"=157, "REG_MAC_WUOFFLONG"=158, "REG_MAC_CLKRECCTRL"=159, "REG_HK_MODE_P2"=162, "REG_MAC_ANTTUNERES1"=164, "REG_MAC_ANTTUNERES2"=165, "REG_INTERFACE_MODE_TEST"=171, "REG_TXRXBUFF_BOTH_P2"=172, "REG_TXRXBUFF_P2"=173, "REG_IRQ_RAWSTATUS1_P2"=174, "REG_MAC_TXIFSTATUS1"=176, "REG_MAC_TXIFSTATUS2"=177, "REG_IRQ_RAWSTATUS2_P2"=178, "REG_MAC_TXIFRAMPDELAY"=179, "REG_MAC_TXIFRAMPSLOPE"=180, "REG_MAX_TXIFRAMP"=181, "REG_IRQ_STATUS1_P2"=182, "REG_IRQ_STATUS2_P2"=183, "REG_IRQ_AUXSTATUS_P2"=184, "REG_MAC_UNLOCK"=188, "REG_MAC_TXIFFREQ"=190, "REG_WAKEUP_TESTCTRL1"=192, "REG_WAKEUP_RX_EN_CNT"=193, "REG_WAKEUP_TESTENABLES"=194, "REG_WAKEUP_DTBI_CTRL"=195, "REG_WAKEUP_DTBO_CTRL"=196, "REG_WAKEUP_TESTIOBUFTEST"=197, "REG_WAKEUP_WK_RX_TESTCTRL1"=198, "REG_WAKEUP_WK_RX_TESTCTRL2"=199, "REG_WAKEUP_SENS_SEQUENCE_CTRL"=200, "REG_WAKEUP_LNABIAS"=201, "REG_WAKEUP_DET_TH_TRIM1"=202, "REG_WAKEUP_LNABIAS_NOM1"=203, "REG_WAKEUP_RX_TSHORT_TRIM1"=204, "REG_WAKEUP_LNABIAS_NOM2"=205, "REG_WAKEUP_RX_TLONG_TRIM1"=206, "REG_WAKEUP_LNA_NEGRTRIM_NOM1"=207, "REG_WAKEUP_RX_TBURST_TRIM1"=208, "REG_WAKEUP_RX_LNA_NEGRTRIM_NOM2"=209, "REG_WAKEUP_RX_BB_G_BW_SEL1"=210, "REG_WAKEUP_WK_RX_DET_IOSTRIM1"=212, "REG_WAKEUP_WK_RX_CTRL2"=214, "REG_WAKEUP_WK_RX_RSSIVOSTRIM"=215, "REG_WAKEUP_LNANEGR_EFF"=216, "REG_WAKEUP_XOSU_FAST"=217, "REG_WAKEUP_STROSCPWIDTH1"=218, "REG_WAKEUP_STROSCPERIOD1"=220, "REG_WAKEUP_STROSCPERIOD2"=221, "REG_WAKEUP_WK_RX_LNA_NEGRTRIM1"=222, "REG_RF_TXTESTENABLE"=224, "REG_RF_TXIFTESTMODE"=225, "REG_RF_RXTESTENABLE"=226, "REG_RF_RXIFTESTCTRL1"=227, "REG_RF_RXIFTESTCTRL2"=228, "REG_RF_RXIFTESTCTRL3"=229, "REG_RF_SYNTH_TESTCTRL1"=230, "REG_RF_SYNTH_TESTCTRL2"=231, "REG_RF_SYNTH_TESTCTRL3"=232, "REG_RF_ADCTEST1"=237, "REG_RF_ADCTEST2"=238, "REG_RF_TXMIXER_IOSTRIM_LOW_IP"=240, "REG_RF_TXMIXER_IOSTRIM_LOW_IN"=241, "REG_RF_TXMIXER_ISOTRIM_LOW_QP"=242, "REG_RF_TXMIXER_IOSTRIM_LOW_QN"=243, "REG_RF_SYNTH_KPD"=244, "REG_RF_SYNTH_LOLEV"=245, "REG_RF_TXRFPWRTUNEANTSET"=246, "REG_RF_TXPD_GAIN_CTRL"=247, "REG_RF_SYNTH_STARTUP"=248, "REG_RF_TXRFANTTUNE_TXMODE"=249, "REG_RF_TXRFANTTUNE_RXMODE"=250, "REG_RF_RXRFANTTUNE_TXMODE"=251, "REG_RF_RXRFANTTUNE_RXMODE"=252, "REG_ANTMATCH1"=253, "REG_ANTMATCH2"=254, "REG_REVISION_P2"=255] ("Register")
            n14 = call "MICSD Set Register.vi"("Execute on Remote?(F)"=w69, "error in (no error)"=w83, "Data"=u8 29, "Address"=w81, "VISA Resource Name"=w84) -> ("error out"=w85:errorcluster, "dup VISA Resource Name"=w86:refnum<visa-resource-name>)  [unwired: 5 in]
            n15 = call "MICSD Set Register.vi"("Execute on Remote?(F)"=w69, "error in (no error)"=w85, "Data"=u8 31, "Address"=w81, "VISA Resource Name"=w86) -> ("error out"=w80:errorcluster, "dup VISA Resource Name"=w77:refnum<visa-resource-name>)  [unwired: 5 in]
            n16 = call "Simple Wait.vi"("mS"=u32 20, "error in"=w80) -> ("error out"=w78:errorcluster)  [unwired: 12 in, 1 out]
            n17 = call "MICSD Get Register.vi"("Execute on Remote?(F)"=w69, "error in (no error)"=w78, "Address"=w76, "VISA Resource Name"=w77) -> ("error out"=w74:errorcluster, "Data"=w75:u8, "dup VISA Resource Name"=w73:refnum<visa-resource-name>)  [unwired: 5 in]
            n18 = To Long Integer(number=w75) -> (32bit integer=w70:i32)
            n19 = Subtract(x=w70, y=32) -> (x-y=w72:i32)
          }
          n20 = Add Array Elements(numeric array=w63) -> (sum=w62:i32)
          n21 = Quotient & Remainder(x=w62, y=w61) -> (floor(x/y)=w59:i32)  [unwired: 1 out]
        }
      }
      n22 = call "MICSD Get Register.vi"("Execute on Remote?(F)"=w10, "error in (no error)"=w32, "Address"=w33, "VISA Resource Name"=w31) -> ("error out"=w37:errorcluster, "Data"=w36:u8, "dup VISA Resource Name"=w38:refnum<visa-resource-name>)  [unwired: 5 in]
      n23 = And(x=u8 191 ("Data"), y=w36) -> (x .and. y?=w35:u8)
      n24 = call "MICSD Set Register.vi"("Execute on Remote?(F)"=w10, "error in (no error)"=w37, "Data"=w35, "Address"=w33, "VISA Resource Name"=w38) -> ("error out"=w14:errorcluster, "dup VISA Resource Name"=w13:refnum<visa-resource-name>)  [unwired: 5 in]
    }
    frame Error {
    }
  }
  "dup VISA Resource Name" <- w5
  "error out" <- w6
  "Wakeup RSSI" <- w1
